vi "QMH_Tester_rev2.vi"() -> ()   [LabVIEW 2024]
doc: "Demonstrates the fundamentals of the Queued Message Handler design pattern in LabVIEW. A queued message handler, in its simplest form, is composed of two loops. The Event Handling Loop responds to user interface events by enqueuing \"messages\" on a message queue. These messages are dequeued in the Message Handling Loop. Note that the Message Handling Loop is also capable of sending messages to itself."
uses:
  Controls/Control_Stop.ctl
  Controls/Control_Unitherm Connect Disconnect Bool.ctl
  Controls/Control_M4X Connect Disconnect Bool.ctl
  Controls/Control_Fornax Connect Disconnect Bool.ctl
  Controls/Control_Unitherm Set Load Numeric.ctl
  Controls/Control_Unitherm Set Load Bool.ctl
  Controls/Control_Unitherm VISA Resource.ctl
  Controls/Control_Unitherm Clear Load Bool.ctl
  Controls/Control_PXI-7854R Connect Disconnect Bool.ctl
  Controls/Control_PXI-7854R 75kHz Bool.ctl
  Controls/Control_PXI-7854R uSec Off Numeric.ctl
  Controls/Control_PXI-7854R uSec On Numeric.ctl
  Controls/Control_PXI-7854R Resource.ctl
  Controls/Control_PXI-7854R Set Config Bool.ctl
  Controls/Control_PXI-7854R Set Config Enum.ctl
  Controls/Control_M4X Read Current Bool.ctl
  Controls/Control_Log Bool.ctl
  Controls/Control_Fornax Ligasure Activate Port Bool.ctl
  Controls/Control_Fornax Bipolar Activate Port Bool.ctl
  Controls/Control_Fornax Bipolar Decrease Power.ctl
  Controls/Control_Fornax Bipolar Increase Power.ctl
  Controls/Control_Fornax Bipolar Enum.ctl
  Controls/Control_Fornax Mono1 Cut Activate Port Bool.ctl
  Controls/Control_Fornax Mono1 Cut Enum.ctl
  Controls/Control_Fornax Mono1 Cut Increase Power.ctl
  Controls/Control_Fornax Mono1 Cut Decrease Power.ctl
  Controls/Control_Fornax Mono1 Coag Enum.ctl
  Controls/Control_Fornax Mono1 Coag Activate Port Bool.ctl
  Controls/Control_Fornax Mono1 Coag Increase Power.ctl
  Controls/Control_Fornax Mono1 Coag Decrease Power.ctl
  Controls/Control_Fornax Mono2 Cut Activate Port Bool.ctl
  Controls/Control_Fornax Mono2 Cut Increase Power.ctl
  Controls/Control_Fornax Mono2 Cut Decrease Power.ctl
  Controls/Control_Fornax Mono2 Cut Enum.ctl
  Controls/Control_Fornax Mono2 Coag Activate Port Bool.ctl
  Controls/Control_Fornax Mono2 Coag Enum.ctl
  Controls/Control_Fornax Mono2 Coag Increase Power.ctl
  Controls/Control_Fornax Mono2 Coag Decrease Power.ctl
  NI Online Practice/CLD Practice/cld_success_package/Preparation_Materials/CLD 6/CLD 6 CSV file enum.ctl
  Controls/Control_Semi-Auto 2-D Array.ctl
  Controls/Control_Fornax Mono1 Cut Power Indicator.ctl
  Controls/Control_Fornax Mono1 Coag Power Indicator.ctl
  Controls/Control_Fornax Mono2 Cut Power Indicator.ctl
  Controls/Control_Fornax Mono2 Coag Power Indicator.ctl
  Controls/Control_Fornax Bipolar Power Indicator.ctl
  Controls/Control_Semi-Auto Cluster Array.ctl
  Controls/Control_Semi-Auto Cluster.ctl
  Controls/Control_Semi-Auto Unitherm Load.ctl
  Controls/Control_Semi-Auto Port.ctl
  Controls/Control_Semi-Auto Mode.ctl
  Controls/Control_Semi-Auto Power Level.ctl
  Controls/Control_Semi-Auto Activation Duration.ctl
  Controls/Control_Footswitch Resource Name.ctl
  Controls/Control_Semi-Auto Cluster Array 2.ctl
  Controls/Control_Semi-Auto Cluster 2.ctl
  Controls/Control_Semi-Auto 2 Activation Method.ctl
  Controls/QMH Fundamentals - Message Cluster.ctl
  Controls/Config_Stop Notifier Enum.ctl
  Controls/Control_Log Cluster.ctl
  Controls/Control_Log Time.ctl
  Controls/Control_Log Waveform Cluster - Current.ctl
  Controls/Control_Log Analysis Cluster - Current.ctl
  Controls/Control_Log Activation Settings Cluster.ctl
  Controls/Control_Log Unitherm Load.ctl
  Controls/Control_Log Port.ctl
  Controls/Control_Log Mode.ctl
  Controls/Control_Log Power Level.ctl
  Controls/Control_Log Waveform Cluster - Diff Voltage.ctl
  Controls/Control_Log Analysis Cluster - Diff Voltage.ctl
  Controls/Control_Log Loop Cluster.ctl
  Controls/Control_Log TDMS Filename.ctl
  Controls/Control_Log t0.ctl
  Controls/Control_Serial Number.ctl
  Controls/Control_Message Handling Cluster.ctl
  Controls/Control_M4X Connection.ctl
  Controls/Control_PXI-7854R FPGA Reference.ctl
  Controls/Control_Config Cluster.ctl
  Controls/Control_Config Unitherm Port.ctl
  Controls/Control_Config Simulate Values.ctl
  Controls/Control_Config Fornax Connect Attempts.ctl
  Controls/Control_Log Queue.ctl
  Controls/Control_Log Flag.ctl
  Controls/Control_Log Port Mode Cluster.ctl
  Controls/Control_Indicator Cluster.ctl
  Controls/Control_Log Power Level Cluster.ctl
  Controls/Control_Log Mono1 Cut Power.ctl
  Controls/Control_Log Mono1 Coag Power.ctl
  Controls/Control_Log Mono2 Cut Power.ctl
  Controls/Control_Log Mono2 Coag Power.ctl
  Controls/Control_Log Bipolar Power.ctl
  Controls/Control_Footswitch Reset Device Bool.ctl
  <instrlib>/niSwitch/niSwitch.llb/niSwitch Topologies.ctl
  Controls/Control_Footswitch Simulate Bool.ctl
  Controls/Control_Unitherm Connect Disconnect Cluster.ctl
  Controls/Control_PXI-7854R Connect Disconnect Cluster.ctl
  Controls/Control_PXI-7854R Set Config Cluster.ctl
  Controls/Control_Auto Set Power Cluster.ctl
  VIs/Abort Auto Test Global.vi
  <vilib>/Utility/error.llb/Error Cluster From Error Code.vi
  <vilib>/ErrorRing/Error Ring.xnode
panel:
  in  "Stop Button":bool
  out "Display Message":string="\"Stop\" button pressed"
  out "Array":T1(array[cluster])
  out "Logging?":bool
  in  "Log?":T2
  out "Fornax Connected?":bool
  out "Unitherm Connected?":bool
  out "M4X Connected?":bool
  out "PXI-7854R Connected?":bool
  in  "Stop":T3
  out "Data":waveform(dbl)[](graph)
  in  "Tab Control":T4(tab)=enum."Semi-Auto"
  out "Mono2 - Coag Power":T5
  out "Mono2 - Cut Power":T6
  out "Mono1 - Coag Power":T7
  out "Mono1 - Cut Power":T8
  in  "Ligasure Activate":T9
  in  "Bipolar Activate":T10
  in  "Bipolar minus":T11
  in  "Bipolar plus":T12
  in  "Bipolar Enum":T13
  in  "Mono1 Cut Activate":T14
  in  "Mono1 Cut Enum":T15
  in  "Mono1 Cut plus":T16
  in  "Mono1 Cut minus":T17
  in  "Mono1 Coag Enum":T18=enum."Spray"
  in  "Mono1 Coag Activate":T19
  in  "Mono1 Coag plus":T20
  in  "Mono1 Coag minus":T21
  in  "Mono2 Cut Activate":T22
  in  "Mono2 Cut plus":T23
  in  "Mono2 Cut minus":T24
  in  "Mono2 Cut Enum":T25
  in  "Mono2 Coag Activate":T26
  in  "Mono2 Coag Enum":T27=enum."Spray"
  in  "Mono2 Coag plus":T28
  in  "Mono2 Coag minus":T29
  out "Bipolar Power":T30
  in  "Unitherm Connect/Disconnect":T31=TRUE
  in  "Load (Ohms)":T32
  in  "Set Load":T33
  in  "Unitherm Refnum in":T34="COM4"
  in  "Clear Load":T35
  in  "7854 Connect/Disconnect":T36=TRUE
  in  "75kHz":T37=TRUE
  in  "uSec Off":T38=6
  in  "uSec On":T39=7
  in  "resource name":T40="PXI1Slot6" caption="RIO Device"
  in  "7854 Set Config":T41
  in  "7854 Config Enum":T42=enum."Off"
  in  "M4X Connect/Disconnect":T43=TRUE
  in  "Fornax Connect/Disconnect":T44=TRUE
  in  "Read Current":T45
  in  "Abort Auto Test":bool
  in  "Update Semi-Auto":bool
  in  "Read/ Write":T46
  in  "Path":path=path "C:/Users/yearon2/OneDrive - Medtronic PLC/LV2015/LT10 Generator Sandbox/FT10_rev2/Semi-Auto Commands.csv"
  out "Semi-Auto 2-D Array out":T47
  in  "Run Semi-Auto Commands":bool
  in  "Semi-Auto Cluster in":T48 {"Power Level" format="%.1f"}
  out "Set Load Case":string="False Case"
  in  "Mono1 Cut - Handswitch":bool
  in  "Mono1 Coag - Handswitch":bool
  in  "Mono2 Triverse Tab":enum32{"Mono 2 - 2 Button", "Mono 2 - Triverse"}(tab)
  in  "Mono2 Cut - Handswitch":bool
  in  "Mono2 Coag - Handswitch":bool
  in  "Triverse Slide":i8(slide) scale=1.0..5.0
  in  "Mono2 Triverse - Handswitch Seal":bool
  in  "Mono2 Triverse - Handswitch Cut":bool
  in  "Mono2 Triverse - Handswitch Coag":bool
  in  "Ligasure - Coag Footswitch":bool
  in  "Ligasure - Cut Footswitch":bool
  in  "Ligasure - Seal Footswitch":bool
  in  "Ligasure - Bipolar Footswitch":bool
  in  "Mono1 Cut - Footswitch":bool
  in  "Mono1 Coag - Footswitch":bool
  in  "Mono2 Cut - Footswitch":bool
  in  "Mono2 Coag - Footswitch":bool
  in  "Bipolar - Footswitch":bool
  in  "Mono2 Triverse - Footswitch":bool
  in  "PXI-2565 resource name":T55="PXI1Slot7" caption="resource name"
  out "Connected?":bool
  in  "Path 2":path=path "C:/Users/yearon2/OneDrive - Medtronic PLC/LV2024/LT10 Generator Sandbox/FT10_rev2/Semi-Auto 2 Commands.csv"
  in  "Run Semi-Auto 2 Commands":bool
  in  "Update Semi-Auto 2":bool
  in  "Read/ Write 2":T46
  out "Semi-Auto 2-D Array out 2":T47
  in  "Semi-Auto 2 Cluster in":T56
  # "Note: If you are creating a LabVIEW application based on the Queued Message Handler design pattern, create a Queued Message Handler project from the File > Create Project dialog."
  # "Bipolar"
  # "Mono2"
  # "Mono1"
  # "Ligasure"
  # "Unitherm"
  # "PXI-7854R"
  # "Fornax"
  # "M4X"
  # "Mono1"
  # "Mono2"
  # "Bipolar"
  # "Ligasure"
  # "Mono1"
  # "Mono2"
  # "Bipolar"
  # "Ligasure"
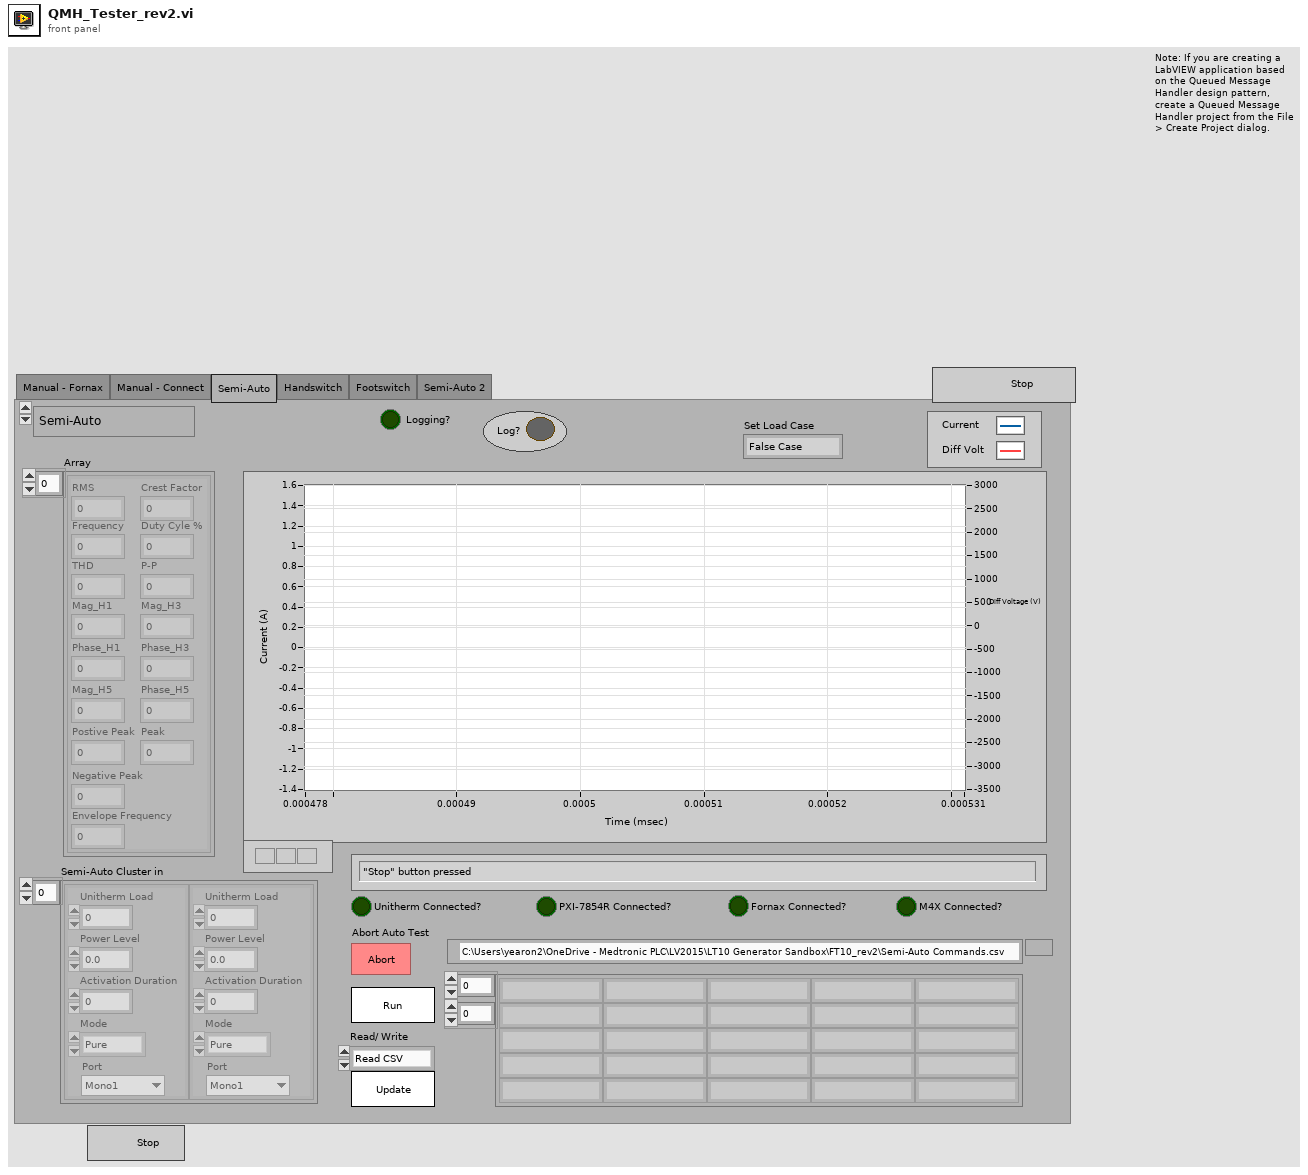
[diagram p1: front panel]
types:
  T1 = cluster{"RMS":dbl, "Envelope Frequency":dbl, "Peak":dbl, "Crest Factor":dbl, "Duty Cyle %":dbl, "P-P":dbl, "Frequency":dbl, "THD":dbl, "Postive Peak":dbl, "Negative Peak":dbl, "Mag_H1":dbl, "Phase_H1":dbl, "Mag_H3":dbl, "Phase_H3":dbl, "Mag_H5":dbl, "Phase_H5":dbl}[]
  T2 = typedef "Control_Log Bool.ctl" = bool
  T3 = typedef "Control_Stop.ctl" = bool
  T4 = enum32{"Manual - Fornax", "Manual - Connect", "Semi-Auto", "Handswitch", "Footswitch", "Semi-Auto 2"}
  T5 = typedef "Control_Fornax Mono2 Coag Power Indicator.ctl" = string
  T6 = typedef "Control_Fornax Mono2 Cut Power Indicator.ctl" = string
  T7 = typedef "Control_Fornax Mono1 Coag Power Indicator.ctl" = string
  T8 = typedef "Control_Fornax Mono1 Cut Power Indicator.ctl" = string
  T9 = typedef "Control_Fornax Ligasure Activate Port Bool.ctl" = bool
  T10 = typedef "Control_Fornax Bipolar Activate Port Bool.ctl" = bool
  T11 = typedef "Control_Fornax Bipolar Decrease Power.ctl" = bool
  T12 = typedef "Control_Fornax Bipolar Increase Power.ctl" = bool
  T13 = typedef "Control_Fornax Bipolar Enum.ctl" = enum16{"Standard", "Macro", "Precision"}
  T14 = typedef "Control_Fornax Mono1 Cut Activate Port Bool.ctl" = bool
  T15 = typedef "Control_Fornax Mono1 Cut Enum.ctl" = enum16{"Pure", "Blend"}
  T16 = typedef "Control_Fornax Mono1 Cut Increase Power.ctl" = bool
  T17 = typedef "Control_Fornax Mono1 Cut Decrease Power.ctl" = bool
  T18 = typedef "Control_Fornax Mono1 Coag Enum.ctl" = enum16{"Fulgerate", "Spray"}
  T19 = typedef "Control_Fornax Mono1 Coag Activate Port Bool.ctl" = bool
  T20 = typedef "Control_Fornax Mono1 Coag Increase Power.ctl" = bool
  T21 = typedef "Control_Fornax Mono1 Coag Decrease Power.ctl" = bool
  T22 = typedef "Control_Fornax Mono2 Cut Activate Port Bool.ctl" = bool
  T23 = typedef "Control_Fornax Mono2 Cut Increase Power.ctl" = bool
  T24 = typedef "Control_Fornax Mono2 Cut Decrease Power.ctl" = bool
  T25 = typedef "Control_Fornax Mono2 Cut Enum.ctl" = enum16{"Pure", "Blend"}
  T26 = typedef "Control_Fornax Mono2 Coag Activate Port Bool.ctl" = bool
  T27 = typedef "Control_Fornax Mono2 Coag Enum.ctl" = enum16{"Fulgerate", "Spray"}
  T28 = typedef "Control_Fornax Mono2 Coag Increase Power.ctl" = bool
  T29 = typedef "Control_Fornax Mono2 Coag Decrease Power.ctl" = bool
  T30 = typedef "Control_Fornax Bipolar Power Indicator.ctl" = string
  T31 = typedef "Control_Unitherm Connect Disconnect Bool.ctl" = bool
  T32 = typedef "Control_Unitherm Set Load Numeric.ctl" = i32
  T33 = typedef "Control_Unitherm Set Load Bool.ctl" = bool
  T34 = typedef "Control_Unitherm VISA Resource.ctl" = refnum<visa-resource-name>
  T35 = typedef "Control_Unitherm Clear Load Bool.ctl" = bool
  T36 = typedef "Control_PXI-7854R Connect Disconnect Bool.ctl" = bool
  T37 = typedef "Control_PXI-7854R 75kHz Bool.ctl" = bool
  T38 = typedef "Control_PXI-7854R uSec Off Numeric.ctl" = u16
  T39 = typedef "Control_PXI-7854R uSec On Numeric.ctl" = u16
  T40 = typedef "Control_PXI-7854R Resource.ctl" = tag
  T41 = typedef "Control_PXI-7854R Set Config Bool.ctl" = bool
  T42 = typedef "Control_PXI-7854R Set Config Enum.ctl" = enum16{"Mono 1", "Mono 2", "BiPolar", "LigaSure", "Off"}
  T43 = typedef "Control_M4X Connect Disconnect Bool.ctl" = bool
  T44 = typedef "Control_Fornax Connect Disconnect Bool.ctl" = bool
  T45 = typedef "Control_M4X Read Current Bool.ctl" = bool
  T46 = typedef "CLD 6 CSV file enum.ctl" = enum16{"Read CSV", "Write CSV"}
  T47 = typedef "Control_Semi-Auto 2-D Array.ctl" = string[][]
  T48 = typedef "Control_Semi-Auto Cluster Array.ctl" = T49[]
  T49 = typedef "Control_Semi-Auto Cluster.ctl" = cluster{"Unitherm Load":T50, "Port":T51, "Mode":T52, "Power Level":T53, "Activation Duration":T54}
  T50 = typedef "Control_Semi-Auto Unitherm Load.ctl" = i32
  T51 = typedef "Control_Semi-Auto Port.ctl" = enum16{"Mono1", "Mono2", "Bipolar", "Ligasure", "Error"}
  T52 = typedef "Control_Semi-Auto Mode.ctl" = enum16{"Pure", "Blend", "Spray", "Fulgerate", "Standard", "Macro", "Precision", "Ligasure", "Error"}
  T53 = typedef "Control_Semi-Auto Power Level.ctl" = dbl
  T54 = typedef "Control_Semi-Auto Activation Duration.ctl" = i32
  T55 = typedef "Control_Footswitch Resource Name.ctl" = refnum<k15>
  T56 = typedef "Control_Semi-Auto Cluster Array 2.ctl" = T57[]
  T57 = typedef "Control_Semi-Auto Cluster 2.ctl" = cluster{"Mode":T52, "Unitherm Load":T50, "Power Level":T53, "Activation Duration":T54, "Port":T51, "Activation Method":T58}
  T58 = typedef "Control_Semi-Auto 2 Activation Method.ctl" = enum16{"Fornax", "Handswitch", "Footswitch"}
  T59 = typedef "Control_Log Loop Cluster.ctl" = cluster{"tdms file out":T60, "t0":T61, "Generator Serial Number in":T62}
  T60 = typedef "Control_Log TDMS Filename.ctl" = refnum<k34>
  T61 = typedef "Control_Log t0.ctl" = string
  T62 = typedef "Control_Serial Number.ctl" = string
  T63 = typedef "Config_Stop Notifier Enum.ctl" = enum16{"Initialize", "Read Notifier", "Notify", "Close"}
  T64 = typedef "Control_Log Cluster.ctl" = cluster{"Log Time":T65, "Log Waveform Cluster - Current":T66, "Log Analysis Cluster - Current":T67, "Log - Activation Settings Cluster":T68, "Log Waveform Cluster - Diff Voltage":T73, "Log Analysis Cluster - Diff Voltage":T74}
  T65 = typedef "Control_Log Time.ctl" = timestamp
  T66 = typedef "Control_Log Waveform Cluster - Current.ctl" = waveform(dbl)
  T67 = typedef "Control_Log Analysis Cluster - Current.ctl" = cluster{"RMS":dbl, "Envelope Frequency":dbl, "Peak":dbl, "Crest Factor":dbl, "Duty Cyle %":dbl, "P-P":dbl, "Frequency":dbl, "THD":dbl, "Postive Peak":dbl, "Negative Peak":dbl, "Mag_H1":dbl, "Phase_H1":dbl, "Mag_H3":dbl, "Phase_H3":dbl, "Mag_H5":dbl, "Phase_H5":dbl}
  T68 = typedef "Control_Log Activation Settings Cluster.ctl" = cluster{"Log - Unitherm Load":T69, "Log - Port":T70, "Log - Mode":T71, "Log - Power Level":T72}
  T69 = typedef "Control_Log Unitherm Load.ctl" = string
  T70 = typedef "Control_Log Port.ctl" = string
  T71 = typedef "Control_Log Mode.ctl" = string
  T72 = typedef "Control_Log Power Level.ctl" = string
  T73 = typedef "Control_Log Waveform Cluster - Diff Voltage.ctl" = waveform(dbl)
  T74 = typedef "Control_Log Analysis Cluster - Diff Voltage.ctl" = cluster{"RMS":dbl, "Envelope Frequency":dbl, "Peak":dbl, "Crest Factor":dbl, "Duty Cyle %":dbl, "P-P":dbl, "Frequency":dbl, "THD":dbl, "Postive Peak":dbl, "Negative Peak":dbl, "Mag_H1":dbl, "Phase_H1":dbl, "Mag_H3":dbl, "Phase_H3":dbl, "Mag_H5":dbl, "Phase_H5":dbl}
  T75 = typedef "QMH Fundamentals - Message Cluster.ctl" = cluster{"Message":string, "Message Data":variant}
  T76 = typedef "Control_Footswitch Simulate Bool.ctl" = bool
  T77 = typedef "niSwitch Topologies.ctl" = string
  T78 = typedef "Control_Footswitch Reset Device Bool.ctl" = bool
  T79 = typedef "Control_Message Handling Cluster.ctl" = cluster{"Fornax Connected?":refnum<vi>, "Unitherm Connected?":refnum<vi>, "M4X Connected?":refnum<vi>, "Unitherm Connect/Disconnect":refnum<vi>, "Fornax Connection":refnum<k5>, "UNITHERM Connection":refnum<visa-resource-name>, "M4X Connection":T80, "FPGA VI Reference Out":T81, "PXI-7854R Connected?":refnum<vi>, "Fornax Connect/Disconnect":refnum<vi>, "7854 Connect/Disconnect":refnum<vi>, "M4X Connect/Disconnect":refnum<vi>, "Config cluster":T82, "Log Queue":T86, "Log Analysis Cluster - Current":T67, "Log Waveform Cluster - Current":T66, "Log Time":T65, "Log Flag":T87, "Log - Activation Settings Cluster":T68, "Log - Port Mode Cluster":T88, "Log Analysis Cluster - Diff Voltage":T74, "Log Waveform Cluster - Diff Voltage":T73, "Indicator Cluster":T89, "Log Power Level Cluster":T90, "Footswitch Cluster":cluster{"PXI-2565 reset device (boolean value)":T78, "topology name":T77, "PXI-2565 simulate (boolean value)":T76, "PXI-2565 resource name":T55}}
  T80 = typedef "Control_M4X Connection.ctl" = u32
  T81 = typedef "Control_PXI-7854R FPGA Reference.ctl" = refnum<k20>
  T82 = typedef "Control_Config Cluster.ctl" = cluster{"Unitherm Port":T83, "Simulate Values":T84, "Fornax Connect Attempts":T85}
  T83 = typedef "Control_Config Unitherm Port.ctl" = string
  T84 = typedef "Control_Config Simulate Values.ctl" = bool
  T85 = typedef "Control_Config Fornax Connect Attempts.ctl" = i32
  T86 = typedef "Control_Log Queue.ctl" = refnum<queue>
  T87 = typedef "Control_Log Flag.ctl" = bool
  T88 = typedef "Control_Log Port Mode Cluster.ctl" = cluster{"Mono1 Cut Enum":T15, "Mono2 Cut Enum":T25, "Mono1 Coag Enum":T18, "Mono2 Coag Enum":T27, "Bipolar Enum":T13}
  T89 = typedef "Control_Indicator Cluster.ctl" = cluster{"Mono1 - Cut Power":refnum<vi>, "Mono1 - Coag Power":refnum<vi>, "Mono2 - Cut Power":refnum<vi>, "Mono2 - Coag Power":refnum<vi>, "Bipolar Power":refnum<vi>, "Mono1 Cut Enum":refnum<vi>, "Mono1 Coag Enum":refnum<vi>, "Mono2 Cut Enum":refnum<vi>, "Mono2 Coag Enum":refnum<vi>, "Bipolar Enum":refnum<vi>}
  T90 = typedef "Control_Log Power Level Cluster.ctl" = cluster{"Log Mono1 Cut Power":T91, "Log Mono1 Coag Power":T92, "Log Mono2 Cut Power":T93, "Log Mono2 Coag Power":T94, "Log Bipolar Power":T95}
  T91 = typedef "Control_Log Mono1 Cut Power.ctl" = string
  T92 = typedef "Control_Log Mono1 Coag Power.ctl" = string
  T93 = typedef "Control_Log Mono2 Cut Power.ctl" = string
  T94 = typedef "Control_Log Mono2 Coag Power.ctl" = string
  T95 = typedef "Control_Log Bipolar Power.ctl" = string
  T96 = typedef "Control_Unitherm Connect Disconnect Cluster.ctl" = cluster{"Unitherm Connect/Disconnect":T31, "Unitherm Refnum in":T34}
  T97 = typedef "Control_PXI-7854R Connect Disconnect Cluster.ctl" = cluster{"PXI-7854R Resource":T40, "75kHz":T37, "uSec Off":T38, "uSec On":T39, "7854 Connect/Disconnect":T36}
  T98 = typedef "Control_PXI-7854R Set Config Cluster.ctl" = cluster{"7854 Config Enum":T42, "7854 Set Config":T41}
  T99 = enum16{"Off", "Mono1 Relay Config", "Mono2 Relay Config", "Bipolar Relay Config", "Ligasure Relay Config", "Handswitch - Mono1 Cut", "Handswitch - Mono1 Coag", "Handswitch - Mono2 Cut", "Handswitch - Mono2 Coag", "Switch to Triverse Mode", "Switch to Mono2 - 2 button Mode", "Triverse Power 1", "Triverse Power 2", "Triverse Power 3", "Triverse Power 4", "Triverse Power 5", "Handswitch - Triverse Seal", "Handswitch - Triverse Cut", "Handswitch - Triverse Coag"}
  T100 = typedef "Control_Auto Set Power Cluster.ctl" = cluster{"Port":T51, "Mode":T52, "Power Level":T53}
  T101 = typedef "Control_Log Filename Cluster.ctl" = cluster{"Current Wvfrm filename":string, "Diff Volt Wvfrm filename":string}
  T102 = typedef "Control_Command Cluster.ctl" = cluster{"Message":string, "Message Data":variant, "Wait Time (ms)":i32}
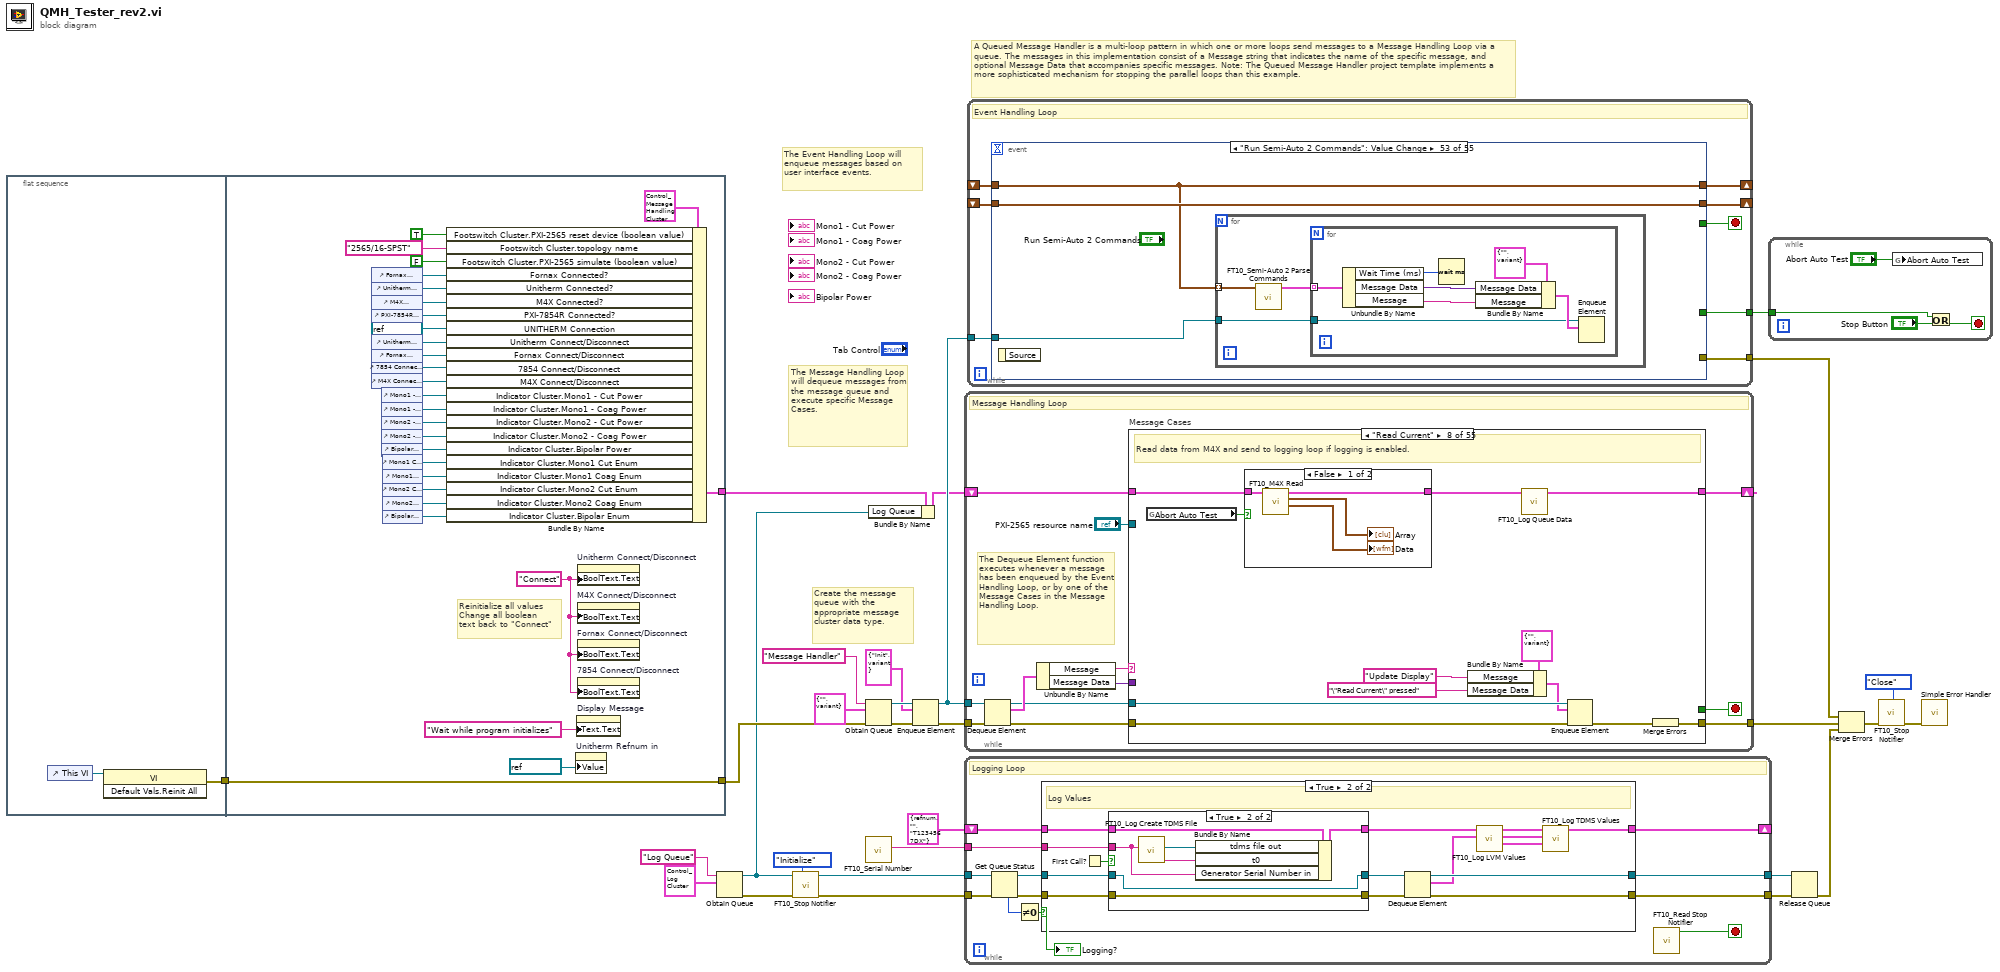
[diagram p0: block diagram]
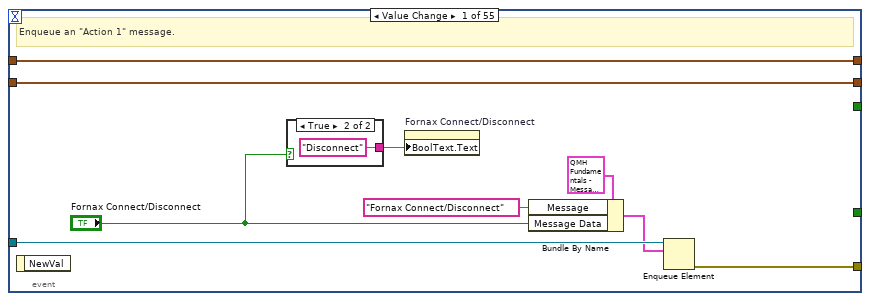
[diagram p4: hidden frame]
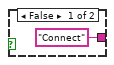
[diagram p5: hidden frame]
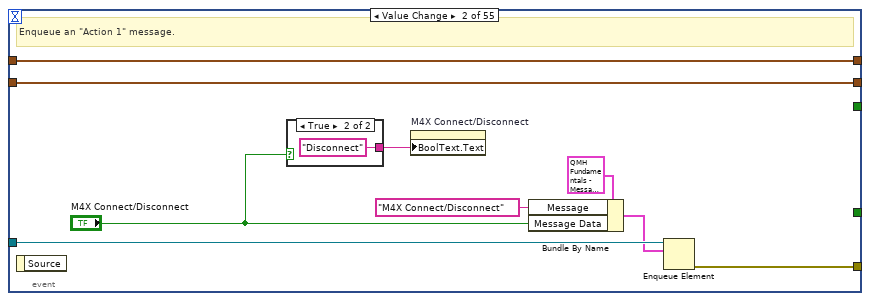
[diagram p6: hidden frame]
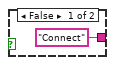
[diagram p7: hidden frame]
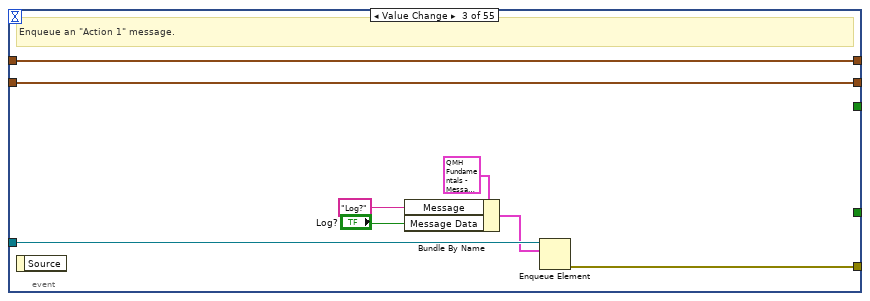
[diagram p8: hidden frame]
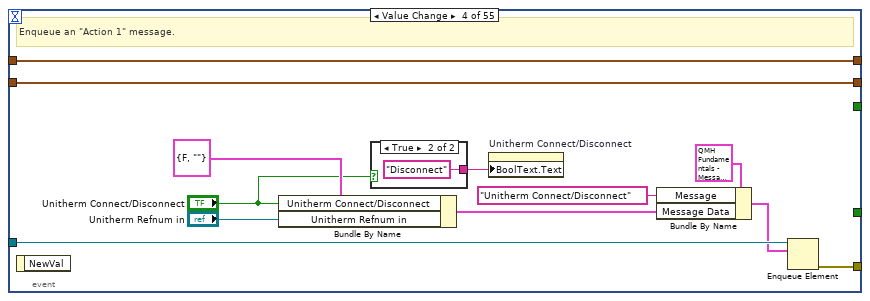
[diagram p9: hidden frame]
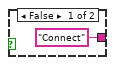
[diagram p10: hidden frame]
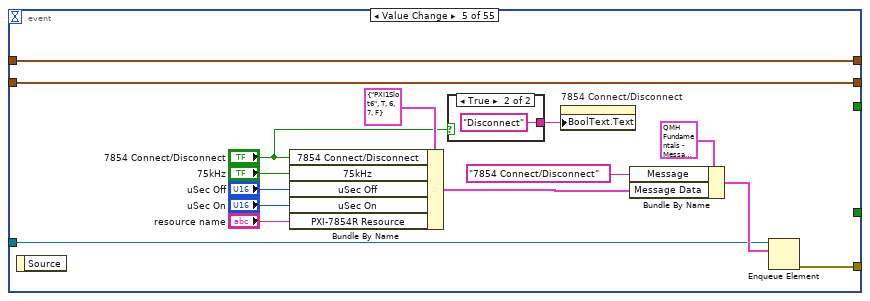
[diagram p11: hidden frame]
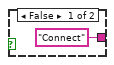
[diagram p12: hidden frame]
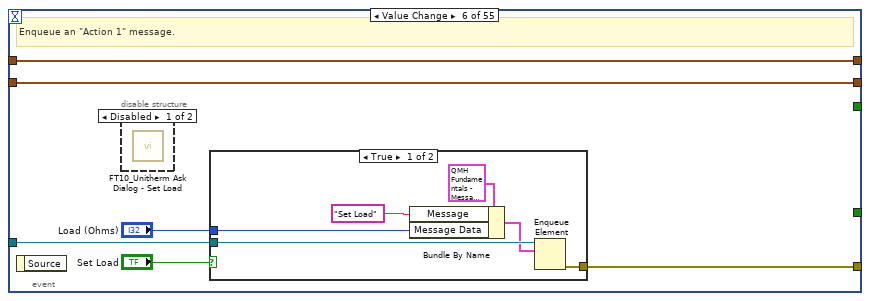
[diagram p13: hidden frame]
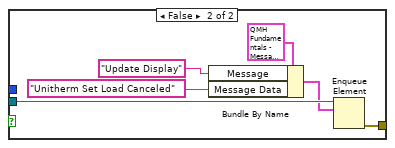
[diagram p15: hidden frame]
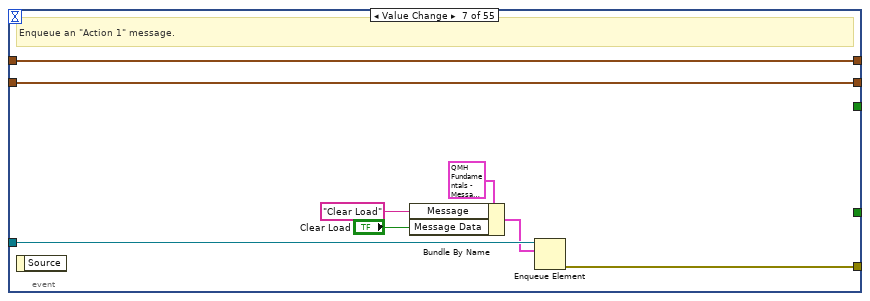
[diagram p16: hidden frame]
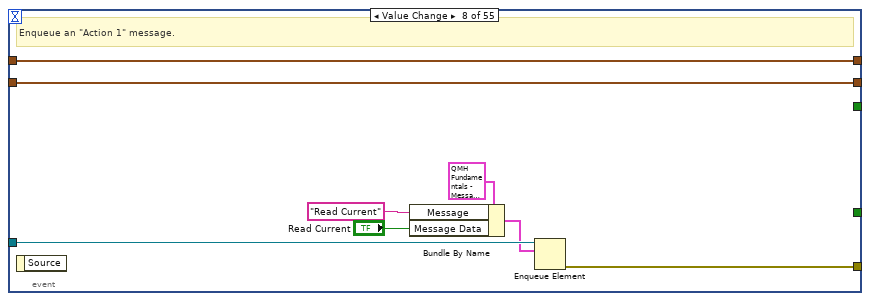
[diagram p17: hidden frame]
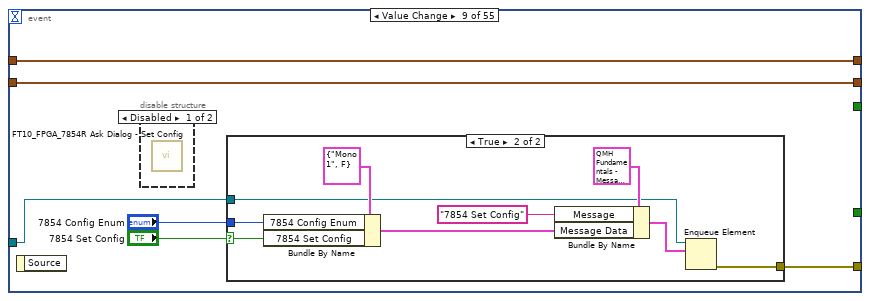
[diagram p18: hidden frame]
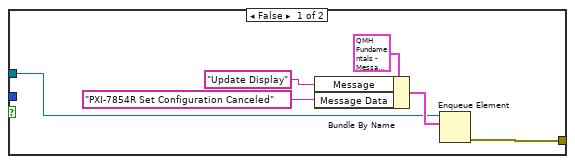
[diagram p20: hidden frame]
diagram:
  # "Create the message queue with the appropriate message cluster data type."
  # "A Queued Message Handler is a multi-loop pattern in which one or more loops send messages to a Message Handling Loop via a queue. The messages in this implementation consist of a Message string that indicates the name of the specific message, and optional Message Data that accompanies specific messages. Note: The Queued Message Handler project template implements a more sophisticated mechanism for stopping the parallel loops than this example."
  # "The Message Handling Loop will dequeue messages from the message queue and execute specific Message Cases."
  # "The Event Handling Loop will enqueue messages based on user interface events."
  n1 = flat-sequence {
    tunnel: [w29] -> w18
    tunnel: [w58] -> w21
    tunnel: w18 -> [w58]
    tunnel: [w48] -> w4
    frame #0 {
      n2 = control-ref of="This VI"() -> (w30:refnum<vi>)
      n3 = invoke class="VI" method="Default Vals.Reinit All"(reference=w30) -> (error out=w29:errorcluster)  [unwired: 2 in, 2 out]
    }
    frame #1 {
      w56 = "Connect" ("Boolean Text.Text")
      # "Reinitialize all values\nChange all boolean\ntext back to \"Connect\""
      n4 = control-ref of="Fornax Connected?"() -> (w34:refnum<vi>)
      n5 = control-ref of="Unitherm Connected?"() -> (w35:refnum<vi>)
      n6 = control-ref of="M4X Connected?"() -> (w36:refnum<vi>)
      n7 = control-ref of="PXI-7854R Connected?"() -> (w37:refnum<vi>)
      n8 = control-ref of="Unitherm Connect/Disconnect"() -> (w39:refnum<vi>)
      n9 = control-ref of="Fornax Connect/Disconnect"() -> (w40:refnum<vi>)
      n10 = control-ref of="7854 Connect/Disconnect"() -> (w41:refnum<vi>)
      n11 = control-ref of="M4X Connect/Disconnect"() -> (w42:refnum<vi>)
      n12 = control-ref of="Mono1 - Cut Power"() -> (w53:refnum<vi>)
      n13 = control-ref of="Mono1 - Coag Power"() -> (w52:refnum<vi>)
      n14 = control-ref of="Mono2 - Cut Power"() -> (w51:refnum<vi>)
      n15 = control-ref of="Mono2 - Coag Power"() -> (w50:refnum<vi>)
      n16 = control-ref of="Bipolar Power"() -> (w49:refnum<vi>)
      n17 = control-ref of="Mono1 Cut Enum"() -> (w47:refnum<vi>)
      n18 = control-ref of="Mono1 Coag Enum"() -> (w46:refnum<vi>)
      n19 = control-ref of="Mono2 Cut Enum"() -> (w45:refnum<vi>)
      n20 = control-ref of="Mono2 Coag Enum"() -> (w44:refnum<vi>)
      n21 = control-ref of="Bipolar Enum"() -> (w43:refnum<vi>)
      n22 = Bundle By Name(cluster=T79 {"Fornax Connected?"=refnum, "Unitherm Connected?"=refnum, "M4X Connected?"=refnum, "Unitherm Connect/Disconnect"=refnum, "Fornax Connection"=refnum, "UNITHERM Connection"="", "M4X Connection"=0, "FPGA VI Reference Out"=refnum, "PXI-7854R Connected?"=refnum, "Fornax Connect/Disconnect"=refnum, "7854 Connect/Disconnect"=refnum, "M4X Connect/Disconnect"=refnum, "Config cluster"={"Unitherm Port"="COM4", "Simulate Values"=TRUE, "Fornax Connect Attempts"=0}, "Log Queue"=refnum, "Log Analysis Cluster - Current"={"RMS"=0.0, "Envelope Frequency"=0.0, "Peak"=0.0, "Crest Factor"=0.0, "Duty Cyle %"=0.0, "P-P"=0.0, "Frequency"=0.0, "THD"=0.0, "Postive Peak"=0.0, "Negative Peak"=0.0, "Mag_H1"=0.0, "Phase_H1"=0.0, "Mag_H3"=0.0, "Phase_H3"=0.0, "Mag_H5"=0.0, "Phase_H5"=0.0}, "Log Waveform Cluster - Current"={"t0"=timestamp(0 s since 1904-01-01), "dt"=1.0, "Y"=[]}, "Log Time"=timestamp(0 s since 1904-01-01), "Log Flag"=FALSE, "Log - Activation Settings Cluster"={"Log - Unitherm Load"="", "Log - Port"="", "Log - Mode"="", "Log - Power Level"=""}, "Log - Port Mode Cluster"={"Mono1 Cut Enum"=enum."Pure", "Mono2 Cut Enum"=enum."Pure", "Mono1 Coag Enum"=enum."Spray", "Mono2 Coag Enum"=enum."Spray", "Bipolar Enum"=enum."Standard"}, "Log Analysis Cluster - Diff Voltage"={"RMS"=0.0, "Envelope Frequency"=0.0, "Peak"=0.0, "Crest Factor"=0.0, "Duty Cyle %"=0.0, "P-P"=0.0, "Frequency"=0.0, "THD"=0.0, "Postive Peak"=0.0, "Negative Peak"=0.0, "Mag_H1"=0.0, "Phase_H1"=0.0, "Mag_H3"=0.0, "Phase_H3"=0.0, "Mag_H5"=0.0, "Phase_H5"=0.0}, "Log Waveform Cluster - Diff Voltage"={"t0"=timestamp(0 s since 1904-01-01), "dt"=1.0, "Y"=[]}, "Indicator Cluster"={"Mono1 - Cut Power"=refnum, "Mono1 - Coag Power"=refnum, "Mono2 - Cut Power"=refnum, "Mono2 - Coag Power"=refnum, "Bipolar Power"=refnum, "Mono1 Cut Enum"=refnum, "Mono1 Coag Enum"=refnum, "Mono2 Cut Enum"=refnum, "Mono2 Coag Enum"=refnum, "Bipolar Enum"=refnum}, "Log Power Level Cluster"={"Log Mono1 Cut Power"="", "Log Mono1 Coag Power"="", "Log Mono2 Cut Power"="", "Log Mono2 Coag Power"="", "Log Bipolar Power"=""}, "Footswitch Cluster"={"PXI-2565 reset device (boolean value)"=TRUE, "topology name"="2565/16-SPST", "PXI-2565 simulate (boolean value)"=FALSE, "PXI-2565 resource name"=""}}, "Footswitch Cluster.PXI-2565 reset device (boolean value)"=T78 TRUE, "Footswitch Cluster.topology name"=T77 "2565/16-SPST", "Footswitch Cluster.PXI-2565 simulate (boolean value)"=T76 FALSE, "Fornax Connected?"=w34, "Unitherm Connected?"=w35, "M4X Connected?"=w36, "PXI-7854R Connected?"=w37, "UNITHERM Connection"=refnum<visa-resource-name> "COM4", "Unitherm Connect/Disconnect"=w39, "Fornax Connect/Disconnect"=w40, "7854 Connect/Disconnect"=w41, "M4X Connect/Disconnect"=w42, "Indicator Cluster.Mono1 - Cut Power"=w53, "Indicator Cluster.Mono1 - Coag Power"=w52, "Indicator Cluster.Mono2 - Cut Power"=w51, "Indicator Cluster.Mono2 - Coag Power"=w50, "Indicator Cluster.Bipolar Power"=w49, "Indicator Cluster.Mono1 Cut Enum"=w47, "Indicator Cluster.Mono1 Coag Enum"=w46, "Indicator Cluster.Mono2 Cut Enum"=w45, "Indicator Cluster.Mono2 Coag Enum"=w44, "Indicator Cluster.Bipolar Enum"=w43) -> (w48:T79)
      n23 = property on="Unitherm Refnum in" class="VISAName (strict)"("Value"=refnum<visa-resource-name> "COM4" ("Unitherm Refnum in")) -> ()  [unwired: 2 in, 2 out]
      n24 = property on="Display Message" class="Str"("Text.Text"="Wait while program initializes" ("Display Message")) -> ()  [unwired: 2 in, 2 out]
      n25 = property on="Unitherm Connect/Disconnect" class="Bool (strict)"("BoolText.Text"=w56) -> ()  [unwired: 2 in, 2 out]
      n26 = property on="M4X Connect/Disconnect" class="Bool (strict)"("BoolText.Text"=w56) -> ()  [unwired: 2 in, 2 out]
      n27 = property on="Fornax Connect/Disconnect" class="Bool (strict)"("BoolText.Text"=w56) -> ()  [unwired: 2 in, 2 out]
      n28 = property on="7854 Connect/Disconnect" class="Bool (strict)"("BoolText.Text"=w56) -> ()  [unwired: 2 in, 2 out]
    }
  }
  n29 = Obtain Queue(name (unnamed)="Log Queue", element data type=T64 {"Log Time"=timestamp(0 s since 1904-01-01), "Log Waveform Cluster - Current"={"t0"=timestamp(0 s since 1904-01-01), "dt"=1.0, "Y"=[]}, "Log Analysis Cluster - Current"={"RMS"=0.0, "Envelope Frequency"=0.0, "Peak"=0.0, "Crest Factor"=0.0, "Duty Cyle %"=0.0, "P-P"=0.0, "Frequency"=0.0, "THD"=0.0, "Postive Peak"=0.0, "Negative Peak"=0.0, "Mag_H1"=0.0, "Phase_H1"=0.0, "Mag_H3"=0.0, "Phase_H3"=0.0, "Mag_H5"=0.0, "Phase_H5"=0.0}, "Log - Activation Settings Cluster"={"Log - Unitherm Load"="", "Log - Port"="", "Log - Mode"="", "Log - Power Level"=""}, "Log Waveform Cluster - Diff Voltage"={"t0"=timestamp(0 s since 1904-01-01), "dt"=1.0, "Y"=[]}, "Log Analysis Cluster - Diff Voltage"={"RMS"=0.0, "Envelope Frequency"=0.0, "Peak"=0.0, "Crest Factor"=0.0, "Duty Cyle %"=0.0, "P-P"=0.0, "Frequency"=0.0, "THD"=0.0, "Postive Peak"=0.0, "Negative Peak"=0.0, "Mag_H1"=0.0, "Phase_H1"=0.0, "Mag_H3"=0.0, "Phase_H3"=0.0, "Mag_H5"=0.0, "Phase_H5"=0.0}}) -> (queue out=w11:refnum<queue>, error out=w9:errorcluster)  [unwired: 3 in, 1 out]
  n30 = call "FT10_Stop Notifier.vi"("Selector"=Config_Stop_Notifier_Enum."Initialize", "error in (no error)"=w9) -> ("error out"=w8:errorcluster)  [unwired: 8 in, 1 out]
  n31 = call "FT10_Serial Number.vi"() -> ("Generator Serial Number out"=w2:T62)  [unwired: 11 in]
  n32 = Obtain Queue(name (unnamed)="Message Handler", element data type=T75 {"Message"="", "Message Data"=variant} ("Message Cluster"), error in (no error)=w21) -> (queue out=w24:refnum<queue>, error out=w25:errorcluster)  [unwired: 2 in, 1 out]
  n33 = Bundle By Name(cluster=w4, "Log Queue"=w11) -> (w12:T79)
  n34 = Enqueue Element(queue=w24, element=T75 {"Message"="Init", "Message Data"=variant}, error in (no error)=w25) -> (queue out=w19:refnum<queue>, error out=w23:errorcluster)  [unwired: 1 in, 1 out]
  n35 = while {
    tunnel: w19 -> [w69]
    tunnel: w23 -> [w70]
    tunnel: [w62] -> w28
    shift-right: [w63] -> _
    shift-left: w12 -> [w60]
    stop <- w61 stop-if-true
    # "The Dequeue Element function executes whenever a message has been enqueued by the Event Handling Loop, or by one of the Message Cases in the Message Handling Loop."
    # "Message Handling Loop"
    n36 = Dequeue Element(queue=w69, error in (no error)=w70) -> (queue out=w67:refnum<queue>, element=w68:T75, error out=w66:errorcluster)  [unwired: 1 in, 1 out]
    n37 = Unbundle By Name(w68) -> ("Message"=w65:string, "Message Data"=w64:variant)
    n38 = case "Message Cases" shown="\"Read Current\"" w65 {
      selector: w65 -> [_ _ _ _ _ _ _ _ _ _ _ _ _ _ _ _ _ _ _ _ _ _ _ _ _ _ _ _ _ _ _ _ _ _ _ _ _ _ _ _ _ _ _ _ _ _ _ _ _ _ _ _ _ _ w994]
      tunnel: w67 -> [w83 w100 w119 w148 w167 w195 w210 w222 w230 w267 w288 w303 w318 w333 w348 w363 w373 w390 w407 w424 w441 w458 w478 w495 w512 w538 w559 w580 w601 w622 w643 w664 w685 w706 w727 w739 w749 w759 w769 w779 w789 w799 w809 w819 w829 w845 w868 w891 w914 w937 w954 _ _ w988 _]
      tunnel: w66 -> [w71 w99 w110 w139 w158 w182 w200 w214 w233 w268 w287 w302 w317 w332 w347 w362 w375 w392 w409 w426 w443 w460 w480 w497 w514 w533 w554 w575 w596 w617 w638 w659 w680 w701 w722 w738 w748 w758 w768 w778 w788 w798 w808 w818 w828 w844 w867 w890 w913 w936 w953 w967 w973 w981 w993]
      tunnel: [w84 w101 w120 w149 w168 w188 w204 w216 w234 w269 w286 w301 w316 w331 w346 w361 w376 w393 w410 w427 w444 w461 w481 w498 w515 w540 w561 w582 w603 w624 w645 w666 w687 w708 w729 w737 w747 w757 w767 w777 w787 w797 w807 w817 w827 w843 w866 w889 w912 w935 w952 w967 w970 w978 w993] -> w62
      tunnel: w64 -> [_ w94 w117 w138 w159 w186 _ _ w239 w273 w283 w299 w314 w328 w343 w358 w380 w397 w414 w431 w448 w465 w485 w502 w519 w544 w565 w586 w607 w628 w649 w670 w691 w712 w733 _ _ _ _ _ _ _ _ _ _ w840 w862 w885 w908 w931 w951 w966 w972 _ _]
      tunnel: w60 -> [w82 w105 w112 w143 w161 w189 w205 w217 w241 w264 w285 w300 w315 w330 w345 w360 w382 w399 w416 w433 w450 w467 w487 w504 w521 w536 w557 w578 w599 w620 w641 w662 w683 w704 w725 w736 w746 w756 w766 w776 w786 w796 w806 w816 w826 w842 w865 w888 w911 w934 w950 w965 w968 w983 w991]
      tunnel: [w80 w98 w111 w142 w160 w176 w197 w212 w240 w262 w279 w294 w309 w324 w339 w354 w381 w398 w415 w432 w449 w466 w486 w503 w520 w530 w551 w572 w593 w614 w635 w656 w677 w698 w719 w735 w745 w754 w764 w774 w784 w794 w804 w814 w824 w836 w859 w882 w905 w928 w950 w964 w968 w982 w991] -> w63
      tunnel: [_ _ _ _ _ _ _ _ _ _ _ _ _ _ _ _ _ _ _ _ _ _ _ _ _ _ _ _ _ _ _ _ _ _ _ _ _ _ _ _ _ _ _ _ _ _ _ _ _ _ _ _ _ TRUE _] -> w61
      tunnel: "PXI-2565 resource name" -> [_ _ _ _ _ _ _ _ _ _ _ _ _ _ _ _ _ _ _ _ _ _ _ _ _ w535 w556 w577 w598 w619 w640 w661 w682 w703 w724 _ _ _ _ _ _ _ _ _ _ _ _ _ _ _ _ _ _ _ _]
      frame "Init" {
        # "Initialize - Create reference for connection indicators. Connect to Fornax, M4X, and Unitherm."
        n39 = call "FT10_Config Parse File.vi"("error in (no error)"=w71, "File Path Control"=path "Config.ini") -> ("error out"=w73:errorcluster, "Config cluster"=w72:T82)  [unwired: 8 in]
        n40 = Bundle By Name(cluster=w82, "Config cluster"=w72) -> (w81:T79)
        n41 = Bundle By Name(cluster=T75 {"Message"="", "Message Data"=variant} ("Message Cluster"), "Message"="Update Display", "Message Data"="Initialize Complete" ("L10n_Action 1 Pressed")) -> (w87:T75)
        n42 = call "FT10_Connect Hardware.vi"("Message Handling Cluster in"=w81, "error in (no error)"=w73) -> ("Message Handling Cluster out"=w80:T79, "Fornax Connected?"=→"Fornax Connected?":bool, "Unitherm Connected?"=→"Unitherm Connected?":bool, "M4X Connected?"=→"M4X Connected?":bool, "PXI-7854R Connected?"=→"PXI-7854R Connected?":bool, "error out"=w79:errorcluster)  [unwired: 8 in]
        n43 = Enqueue Element(queue=w83, element=w87, error in (no error)=w71) -> (error out=w85:errorcluster)  [unwired: 1 in, 2 out]
        n44 = Merge Errors(w79, w85) -> (w84:errorcluster)
      }
      frame "Fornax Connect/Disconnect" {
        # "Connect or disconnect from Fornax."
        n45 = Variant To Data(type=TRUE, Variant=w94) -> (data=w91:bool)  [unwired: 1 in, 1 out]
        n46 = case shown="True" w91 {
          tunnel: ["Fornax Disconnect" ("L10n_Action 1 Pressed") "Fornax Connect" ("L10n_Action 1 Pressed")] -> w90
          frame False {
          }
          frame True {
          }
        }
        n47 = call "FT10_Connect Fornax Handler.vi"("error in (no error)"=w99, "Message Data"=w94, "Message Handling Cluster in"=w105) -> ("error out"=w96:errorcluster, "Fornax Connected?"=w95:bool, "Message Handling Cluster out"=w98:T79)  [unwired: 6 in]
        n48 = Bundle By Name(cluster=T75 {"Message"="", "Message Data"=variant} ("Message Cluster"), "Message Data"=w90, "Message"="Update Display") -> (w103:T75)
        n49 = Enqueue Element(queue=w100, element=w103, error in (no error)=w99) -> (error out=w102:errorcluster)  [unwired: 1 in, 2 out]
        n50 = Unbundle By Name(w98) -> ("Fornax Connected?"=w97:refnum<vi>)
        n51 = property class="Bool (strict)"(reference=w97, "Value"=w95) -> ()  [unwired: 1 in, 2 out]
        n52 = Merge Errors(w96, w102) -> (w101:errorcluster)
      }
      frame "M4X Connect/Disconnect" {
        # "Connect or disconnect from M4X."
        n53 = Variant To Data(type=TRUE, Variant=w117) -> (data=w114:bool)  [unwired: 1 in, 1 out]
        n54 = case shown="True" w114 {
          tunnel: ["M4X Disconnect" ("L10n_Action 1 Pressed") "M4X Connect" ("L10n_Action 1 Pressed")] -> w113
          tunnel: w112 -> [w126 w132]
          tunnel: [w126 w131] -> w111
          tunnel: w110 -> [w125 w130]
          tunnel: [w125 w129] -> w109
          tunnel: [FALSE ("M4X Connected?") w128] -> w108
          frame False {
          }
          frame True {
            n55 = call "FT10_Connect M4X.vi"("error in (no error)"=w130, "reset device"=TRUE, "Board #"=u32 0, "Message Handling Cluster in"=w132) -> ("error out"=w129:errorcluster, "M4X Connected?"=w128:bool, "Message Handling Cluster out"=w131:T79)  [unwired: 4 in, 1 out]
          }
        }
        n56 = Bundle By Name(cluster=T75 {"Message"="", "Message Data"=variant} ("Message Cluster"), "Message Data"=w113, "Message"="Update Display") -> (w122:T75)
        n57 = Enqueue Element(queue=w119, element=w122, error in (no error)=w110) -> (error out=w121:errorcluster)  [unwired: 1 in, 2 out]
        n58 = Unbundle By Name(w111) -> ("M4X Connected?"=w118:refnum<vi>)
        n59 = property class="Bool (strict)"(reference=w118, "Value"=w108) -> ()  [unwired: 1 in, 2 out]
        n60 = Merge Errors(w109, w121) -> (w120:errorcluster)
      }
      frame "Unitherm Connect/Disconnect" {
        # "Connect or disconnect from Unitherm."
        n61 = Variant To Data(type=T96 {"Unitherm Connect/Disconnect"=FALSE, "Unitherm Refnum in"=""}, Variant=w138) -> (data=w145:T96)  [unwired: 1 in, 1 out]
        n62 = Unbundle By Name(w145) -> ("Unitherm Connect/Disconnect"=w136:T31)
        n63 = call "FT10_Connect Unitherm Handler.vi"("error in (no error)"=w139, "Message Data"=w138, "Message Handling Cluster in"=w143) -> ("error out"=w140:errorcluster, "Unitherm Connected?"=w141:bool, "Message Handling Cluster out"=w142:T79)  [unwired: 6 in]
        n64 = case shown="False" w136 {
          tunnel: ["Unitherm Disconnect" ("L10n_Action 1 Pressed") "Unitherm Connect" ("L10n_Action 1 Pressed")] -> w144
          frame False {
          }
          frame True {
          }
        }
        n65 = Unbundle By Name(w142) -> ("Unitherm Connected?"=w147:refnum<vi>)
        n66 = Bundle By Name(cluster=T75 {"Message"="", "Message Data"=variant} ("Message Cluster"), "Message Data"=w144, "Message"="Update Display") -> (w151:T75)
        n67 = Enqueue Element(queue=w148, element=w151, error in (no error)=w139) -> (error out=w150:errorcluster)  [unwired: 1 in, 2 out]
        n68 = property class="Bool (strict)"(reference=w147, "Value"=w141) -> ()  [unwired: 1 in, 2 out]
        n69 = Merge Errors(w140, w150) -> (w149:errorcluster)
      }
      frame "7854 Connect/Disconnect" {
        # "Connect or disconnect from Unitherm."
        n70 = Variant To Data(type=T97 {"PXI-7854R Resource"="PXI1Slot6", "75kHz"=TRUE, "uSec Off"=6, "uSec On"=7, "7854 Connect/Disconnect"=FALSE}, Variant=w159) -> (data=w164:T97)  [unwired: 1 in, 1 out]
        n71 = Unbundle By Name(w164) -> ("7854 Connect/Disconnect"=w162:T36)
        n72 = case shown="False" w162 {
          tunnel: ["PXI-7854R Disconnected" ("L10n_Action 1 Pressed") "PXI-7854R Connected" ("L10n_Action 1 Pressed")] -> w163
          frame False {
          }
          frame True {
          }
        }
        n73 = call "FT10_Connect FPGA_7854R Handler.vi"("error in"=w158, "Message Data"=w159, "Message Handling Cluster in"=w161) -> ("error out"=w157:errorcluster, "PXI-7854R Connected?"=w156:bool, "Message Handling Cluster out"=w160:T79)  [unwired: 6 in]
        n74 = Unbundle By Name(w160) -> ("PXI-7854R Connected?"=w166:refnum<vi>)
        n75 = Bundle By Name(cluster=T75 {"Message"="", "Message Data"=variant} ("Message Cluster"), "Message Data"=w163, "Message"="Update Display") -> (w170:T75)
        n76 = Enqueue Element(queue=w167, element=w170, error in (no error)=w158) -> (error out=w169:errorcluster)  [unwired: 1 in, 2 out]
        n77 = property class="Bool (strict)"(reference=w166, "Value"=w156) -> ()  [unwired: 1 in, 2 out]
        n78 = Merge Errors(w157, w169) -> (w168:errorcluster)
      }
      frame "Set Load" {
        # "Adjust the Impedance of the Unitherm."
        n79 = Variant To Data(type=0 ("Load (Ohms)"), Variant=w186) -> (data=w178:i32)  [unwired: 1 in, 1 out]
        n80 = Number To Decimal String(number=w178) -> (decimal integer string=w180:string)  [unwired: 1 in]
        n81 = Unbundle By Name(w189) -> ("UNITHERM Connection"=w185:refnum<visa-resource-name>)
        n82 = Concatenate Strings("Unitherm Load set to " ("L10n_Action 1 Pressed"), w180, " Ohms" ("string")) -> (w181:string)
        n83 = call "FT10_Unitherm Set Load.vi"("error in (no error)"=w182, "Load Impedance in"=w178, "VISA Refnum in"=w185) -> ("error out"=w183:errorcluster, "Load Impedance out"=w175:i32, "VISA Refnum out"=w184:refnum<visa-resource-name>, "Set Load Case"=→"Set Load Case":string)  [unwired: 5 in]
        n84 = Bundle By Name(cluster=T75 {"Message"="", "Message Data"=variant} ("Message Cluster"), "Message"="Update Display", "Message Data"=w181) -> (w191:T75)
        n85 = Bundle By Name(cluster=w189, "UNITHERM Connection"=w184) -> (w177:T79)
        n86 = Enqueue Element(queue=w195, element=w191, error in (no error)=w182) -> (error out=w194:errorcluster)  [unwired: 1 in, 2 out]
        n87 = Merge Errors(w183, w194) -> (w188:errorcluster)
        n88 = call "FT10_Log Update Unitherm Load Value.vi"("Load Impedance in"=w175, "Message Handling Cluster in"=w177) -> ("Message Handling Cluster out"=w176:T79)  [unwired: 9 in]
      }
      frame "Clear Load" {
        # "Adjust the Impedance of the Unitherm."
        n89 = Unbundle By Name(w205) -> ("UNITHERM Connection"=w202:refnum<visa-resource-name>)
        n90 = call "FT10_Unitherm Clear Load.vi"("error in (no error)"=w200, "VISA Refnum in"=w202) -> ("error out"=w199:errorcluster, "Load Impedance out"=w196:i32, "VISA Refnum out"=w201:refnum<visa-resource-name>)  [unwired: 7 in]
        n91 = Bundle By Name(cluster=T75 {"Message"="", "Message Data"=variant} ("Message Cluster"), "Message"="Update Display", "Message Data"="Unitherm Load Cleared" ("L10n_Action 1 Pressed")) -> (w206:T75)
        n92 = Bundle By Name(cluster=w205, "UNITHERM Connection"=w201) -> (w198:T79)
        n93 = Enqueue Element(queue=w210, element=w206, error in (no error)=w200) -> (error out=w209:errorcluster)  [unwired: 1 in, 2 out]
        n94 = Merge Errors(w199, w209) -> (w204:errorcluster)
        n95 = call "FT10_Log Update Unitherm Load Value.vi"("Load Impedance in"=w196, "Message Handling Cluster in"=w198) -> ("Message Handling Cluster out"=w197:T79)  [unwired: 9 in]
      }
      frame "Read Current" {
        # "Read data from M4X and send to logging loop if logging is enabled."
        n96 = global read "Abort Auto Test Global.vi" "Abort Auto Test"() -> (w211:bool)
        n97 = case shown="False" w211 {
          tunnel: w217 -> [w226 w227]
          tunnel: [w223 w227] -> w213
          frame False {
            n98 = call "FT10_M4X Read.vi"("Message Handling Cluster in"=w226) -> ("Waveform Array"=→"Data":waveform(dbl)[], "Analysis Cluster Array"=→"Array":T1, "Message Handling Cluster out"=w223:T79)  [unwired: 8 in]
          }
          frame True {
          }
        }
        n99 = Bundle By Name(cluster=T75 {"Message"="", "Message Data"=variant} ("Message Cluster"), "Message"="Update Display", "Message Data"="\"Read Current\" pressed" ("L10n_Action 1 Pressed")) -> (w218:T75)
        n100 = call "FT10_Log Queue Data.vi"("Message Handling Cluster in"=w213) -> ("Message Handling Cluster out"=w212:T79)  [unwired: 10 in]
        n101 = Enqueue Element(queue=w222, element=w218, error in (no error)=w214) -> (error out=w221:errorcluster)  [unwired: 1 in, 2 out]
        n102 = Merge Errors(w221) -> (w216:errorcluster)
      }
      frame "7854 Set Config" {
        n103 = global read "Abort Auto Test Global.vi" "Abort Auto Test"() -> (w229:bool)
        n104 = Variant To Data(type=T98 {"7854 Config Enum"=enum."Mono 1", "7854 Set Config"=FALSE}, Variant=w239) -> (data=w242:T98)  [unwired: 1 in, 1 out]
        n105 = Unbundle By Name(w242) -> ("7854 Config Enum"=w228:T42)
        n106 = case shown="False" w229 {
          tunnel: w241 -> [w249 w259]
          tunnel: [w248 w258] -> w240
          tunnel: w228 -> [w244 _]
          frame False {
            n107 = Unbundle By Name(w249) -> ("FPGA VI Reference Out"=w247:T81)
            n108 = case shown="\"BiPolar\"" w244 {
              tunnel: [T99."Off" ("Update Config Enum") T99."Mono1 Relay Config" ("Update Config Enum") T99."Mono2 Relay Config" ("Update Config Enum") T99."Bipolar Relay Config" ("Update Config Enum") T99."Ligasure Relay Config" ("Update Config Enum")] -> w245
              frame "Off" {
              }
              frame "Mono 1" {
              }
              frame "Mono 2" {
              }
              frame "BiPolar" {
              }
              frame "LigaSure" {
              }
            }
            n109 = call "FT10_FPGA_7854R Set Relay Config.vi"("Update Config Enum"=w245, "Refnum in"=w247) -> ("Refnum out"=w246:T81)  [unwired: 9 in]
            n110 = Bundle By Name(cluster=w249, "FPGA VI Reference Out"=w246) -> (w248:T79)
          }
          frame True {
            n111 = Unbundle By Name(w259) -> ("FPGA VI Reference Out"=w256:T81)
            n112 = call "FT10_FPGA_7854R Set Relay Config.vi"("Update Config Enum"=T99."Off", "Refnum in"=w256) -> ("Refnum out"=w257:T81)  [unwired: 9 in]
            n113 = Bundle By Name(cluster=w259, "FPGA VI Reference Out"=w257) -> (w258:T79)
          }
        }
        n114 = call "FT10_FPGA_7854R Set Config.vi"("7854 Config Enum"=w228) -> ("Config string"=w232:string)  [unwired: 7 in, 3 out]
        n115 = Concatenate Strings("PXI-7854R Configuration Set to " ("Display Message"), w232) -> (w231:string)
        n116 = Bundle By Name(cluster=T75 {"Message"="", "Message Data"=variant} ("Message Cluster"), "Message"="Update Display", "Message Data"=w231) -> (w235:T75)
        n117 = Enqueue Element(queue=w230, element=w235, error in (no error)=w233) -> (error out=w234:errorcluster)  [unwired: 1 in, 2 out]
      }
      frame "Auto Set Power" {
        n118 = Variant To Data(type=T100 {"Port"=enum."Mono1", "Mode"=enum."Pure", "Power Level"=0.0}, Variant=w273) -> (data=w263:T100)  [unwired: 1 in, 1 out]
        n119 = global read "Abort Auto Test Global.vi" "Abort Auto Test"() -> (w260:bool)
        n120 = case shown="False" w260 {
          tunnel: w264 -> [w276 w277]
          tunnel: w263 -> [w275 _]
          tunnel: [w274 w277] -> w261
          frame False {
            n121 = call "FT10_Semi-Auto Power Set and Read.vi"("Auto Set Power Cluster in"=w275, "Message Handling Cluster in"=w276) -> ("Message Handling Cluster out"=w274:T79)  [unwired: 8 in, 1 out]
          }
          frame True {
          }
        }
        n122 = call "FT10_Semi-Auto Set Power Display String.vi"("Auto Set Power Cluster"=w263) -> ("Display String"=w265:string)  [unwired: 10 in]
        n123 = Bundle By Name(cluster=T75 {"Message"="", "Message Data"=variant} ("Message Cluster"), "Message"="Update Display", "Message Data"=w265) -> (w270:T75)
        n124 = call "FT10_Fornax Read and Parse.vi"("Message Handling Cluster in"=w261) -> ("Message Handling Cluster out"=w262:T79)  [unwired: 9 in, 1 out]
        n125 = Enqueue Element(queue=w267, element=w270, error in (no error)=w268) -> (error out=w269:errorcluster)  [unwired: 1 in, 2 out]
      }
      frame "Mono1 Cut Activate Port" {
        # "Turn power ON or OFF on MONO1 Cut Port"
        n126 = Variant To Data(type=T14 FALSE ("Mono1 Cut Activate"), Variant=w283) -> (data=w278:T14)  [unwired: 1 in, 1 out]
        n127 = Unbundle By Name(w285) -> ("Fornax Connection"=w282:refnum<k5>)
        n128 = call "FT10_Fornax Mono1 Cut Activate Port Command.vi"("Mono1 Cut Activate"=w278, "TCP Network Connection in"=w282) -> ("TCP Network Connection out"=w281:refnum<k5>)  [unwired: 9 in]
        n129 = Bundle By Name(cluster=w285, "Fornax Connection"=w281) -> (w280:T79)
        n130 = Bundle By Name(cluster=T75 {"Message"="", "Message Data"=variant} ("Message Cluster"), "Message"="Update Display", "Message Data"="\"Mono1 Cut Activate Port\" pressed" ("L10n_Action 1 Pressed")) -> (w290:T75)
        n131 = call "FT10_Log Update Mono1 Cut Log.vi"("Mono1 Cut Activate"=w278, "Message Handling Cluster in"=w280) -> ("Message Handling Cluster out"=w279:T79)  [unwired: 9 in]
        n132 = Enqueue Element(queue=w288, element=w290, error in (no error)=w287) -> (error out=w286:errorcluster)  [unwired: 1 in, 2 out]
      }
      frame "Mono2 Cut Activate Port" {
        # "Turn power ON or OFF on MONO2 Cut Port"
        n133 = Variant To Data(type=T22 FALSE ("Mono2 Cut Activate"), Variant=w299) -> (data=w293:T22)  [unwired: 1 in, 1 out]
        n134 = Unbundle By Name(w300) -> ("Fornax Connection"=w297:refnum<k5>)
        n135 = call "FT10_Fornax Mono2 Cut Activate Port Command.vi"("Mono2 Cut Activate"=w293, "TCP Network Connection in"=w297) -> ("TCP Network Connection out"=w296:refnum<k5>)  [unwired: 9 in]
        n136 = Bundle By Name(cluster=w300, "Fornax Connection"=w296) -> (w295:T79)
        n137 = Bundle By Name(cluster=T75 {"Message"="", "Message Data"=variant} ("Message Cluster"), "Message"="Update Display", "Message Data"="\"Mono2 Cut Activate Port\" pressed" ("L10n_Action 1 Pressed")) -> (w305:T75)
        n138 = call "FT10_Log Update Mono2 Cut Log.vi"("Mono2 Cut Activate"=w293, "Message Handling Cluster in"=w295) -> ("Message Handling Cluster out"=w294:T79)  [unwired: 9 in]
        n139 = Enqueue Element(queue=w303, element=w305, error in (no error)=w302) -> (error out=w301:errorcluster)  [unwired: 1 in, 2 out]
      }
      frame "Mono1 Coag Activate Port" {
        # "Turn power ON or OFF on MONO1 Coag Port"
        n140 = Variant To Data(type=T19 FALSE ("Mono1 Coag Activate"), Variant=w314) -> (data=w308:T19)  [unwired: 1 in, 1 out]
        n141 = Unbundle By Name(w315) -> ("Fornax Connection"=w312:refnum<k5>)
        n142 = call "FT10_Fornax Mono1 Coag Activate Port Command.vi"("Mono1 Coag Activate"=w308, "TCP Network Connection in"=w312) -> ("TCP Network Connection out"=w311:refnum<k5>)  [unwired: 9 in]
        n143 = Bundle By Name(cluster=w315, "Fornax Connection"=w311) -> (w310:T79)
        n144 = Bundle By Name(cluster=T75 {"Message"="", "Message Data"=variant} ("Message Cluster"), "Message"="Update Display", "Message Data"="\"Mono1 Coag Activate Port\" pressed" ("L10n_Action 1 Pressed")) -> (w320:T75)
        n145 = call "FT10_Log Update Mono1 Coag Log.vi"("Mono1 Coag Activate"=w308, "Message Handling Cluster in"=w310) -> ("Message Handling Cluster out"=w309:T79)  [unwired: 9 in]
        n146 = Enqueue Element(queue=w318, element=w320, error in (no error)=w317) -> (error out=w316:errorcluster)  [unwired: 1 in, 2 out]
      }
      frame "Mono2 Coag Activate Port" {
        # "Turn power ON or OFF on MONO2 Coag Port"
        n147 = Variant To Data(type=T26 FALSE ("Mono2 Coag Activate"), Variant=w328) -> (data=w323:T26)  [unwired: 1 in, 1 out]
        n148 = Unbundle By Name(w330) -> ("Fornax Connection"=w327:refnum<k5>)
        n149 = call "FT10_Fornax Mono2 Coag Activate Port Command.vi"("Mono2 Coag Activate"=w323, "TCP Network Connection in"=w327) -> ("TCP Network Connection out"=w326:refnum<k5>)  [unwired: 9 in]
        n150 = Bundle By Name(cluster=w330, "Fornax Connection"=w326) -> (w325:T79)
        n151 = Bundle By Name(cluster=T75 {"Message"="", "Message Data"=variant} ("Message Cluster"), "Message"="Update Display", "Message Data"="\"Mono2 Coag Activate Port\" pressed" ("L10n_Action 1 Pressed")) -> (w335:T75)
        n152 = call "FT10_Log Update Mono2 Coag Log.vi"("Mono2 Coag Activate"=w323, "Message Handling Cluster in"=w325) -> ("Message Handling Cluster out"=w324:T79)  [unwired: 9 in]
        n153 = Enqueue Element(queue=w333, element=w335, error in (no error)=w332) -> (error out=w331:errorcluster)  [unwired: 1 in, 2 out]
      }
      frame "Ligasure Activate Port" {
        # "Turn power ON or OFF on Ligasure Port"
        n154 = Variant To Data(type=T9 FALSE ("Ligasure Activate"), Variant=w343) -> (data=w338:T9)  [unwired: 1 in, 1 out]
        n155 = Unbundle By Name(w345) -> ("Fornax Connection"=w342:refnum<k5>)
        n156 = call "FT10_Fornax Ligasure Activate Port Command.vi"("Ligasure Activate"=w338, "TCP Network Connection in"=w342) -> ("TCP Network Connection out"=w341:refnum<k5>)  [unwired: 9 in]
        n157 = Bundle By Name(cluster=w345, "Fornax Connection"=w341) -> (w340:T79)
        n158 = Bundle By Name(cluster=T75 {"Message"="", "Message Data"=variant} ("Message Cluster"), "Message"="Update Display", "Message Data"="\"Ligasure Activate Port\" pressed" ("L10n_Action 1 Pressed")) -> (w350:T75)
        n159 = call "FT10_Log Update Ligasure Log.vi"("Ligasure Activate"=w338, "Message Handling Cluster in"=w340) -> ("Message Handling Cluster out"=w339:T79)  [unwired: 9 in]
        n160 = Enqueue Element(queue=w348, element=w350, error in (no error)=w347) -> (error out=w346:errorcluster)  [unwired: 1 in, 2 out]
      }
      frame "Bipolar Activate Port" {
        # "Turn power ON or OFF on Bipolar Port"
        n161 = Variant To Data(type=T10 FALSE ("Bipolar Activate"), Variant=w358) -> (data=w353:T10)  [unwired: 1 in, 1 out]
        n162 = Unbundle By Name(w360) -> ("Fornax Connection"=w357:refnum<k5>)
        n163 = call "FT10_Fornax Bipolar Activate Port Command.vi"("Bipolar Activate"=w353, "TCP Network Connection in"=w357) -> ("TCP Network Connection out"=w356:refnum<k5>)  [unwired: 9 in]
        n164 = Bundle By Name(cluster=w360, "Fornax Connection"=w356) -> (w355:T79)
        n165 = Bundle By Name(cluster=T75 {"Message"="", "Message Data"=variant} ("Message Cluster"), "Message"="Update Display", "Message Data"="\"Bipolar Activate Port\" pressed" ("L10n_Action 1 Pressed")) -> (w365:T75)
        n166 = call "FT10_Log Update Bipolar Log.vi"("Bipolar Activate"=w353, "Message Handling Cluster in"=w355) -> ("Message Handling Cluster out"=w354:T79)  [unwired: 9 in]
        n167 = Enqueue Element(queue=w363, element=w365, error in (no error)=w362) -> (error out=w361:errorcluster)  [unwired: 1 in, 2 out]
      }
      frame "Mono1 Cut - Handswitch Activate Port" {
        n168 = Variant To Data(type=TRUE, Variant=w380) -> (data=w371:bool)  [unwired: 1 in, 1 out]
        n169 = case shown="False" w371 {
          tunnel: [T99."Handswitch - Mono1 Cut" ("Update Config Enum") T99."Mono1 Relay Config" ("Update Config Enum")] -> w368
          frame True {
          }
          frame False {
          }
        }
        n170 = Unbundle By Name(w382) -> ("FPGA VI Reference Out"=w370:T81)
        n171 = call "FT10_FPGA_7854R Set Relay Config.vi"("Update Config Enum"=w368, "Refnum in"=w370) -> ("Refnum out"=w369:T81)  [unwired: 9 in]
        n172 = Bundle By Name(cluster=T75 {"Message"="", "Message Data"=variant} ("Message Cluster"), "Message"="Update Display", "Message Data"="Mono1 Cut - Handswitch Activate Port" ("Display Message")) -> (w377:T75)
        n173 = Bundle By Name(cluster=w382, "FPGA VI Reference Out"=w369) -> (w381:T79)
        n174 = Enqueue Element(queue=w373, element=w377, error in (no error)=w375) -> (error out=w376:errorcluster)  [unwired: 1 in, 2 out]
      }
      frame "Mono1 Coag - Handswitch Activate Port" {
        n175 = Variant To Data(type=TRUE, Variant=w397) -> (data=w388:bool)  [unwired: 1 in, 1 out]
        n176 = case shown="True" w388 {
          tunnel: [T99."Handswitch - Mono1 Coag" ("Update Config Enum") T99."Mono1 Relay Config" ("Update Config Enum")] -> w385
          frame True {
          }
          frame False {
          }
        }
        n177 = Unbundle By Name(w399) -> ("FPGA VI Reference Out"=w387:T81)
        n178 = call "FT10_FPGA_7854R Set Relay Config.vi"("Update Config Enum"=w385, "Refnum in"=w387) -> ("Refnum out"=w386:T81)  [unwired: 9 in]
        n179 = Bundle By Name(cluster=T75 {"Message"="", "Message Data"=variant} ("Message Cluster"), "Message"="Update Display", "Message Data"="Mono1 Coag - Handswitch Activate Port" ("Display Message")) -> (w394:T75)
        n180 = Bundle By Name(cluster=w399, "FPGA VI Reference Out"=w386) -> (w398:T79)
        n181 = Enqueue Element(queue=w390, element=w394, error in (no error)=w392) -> (error out=w393:errorcluster)  [unwired: 1 in, 2 out]
      }
      frame "Mono2 Cut - Handswitch Activate Port" {
        n182 = Variant To Data(type=TRUE, Variant=w414) -> (data=w405:bool)  [unwired: 1 in, 1 out]
        n183 = case shown="False" w405 {
          tunnel: [T99."Handswitch - Mono2 Cut" ("Update Config Enum") T99."Mono2 Relay Config" ("Update Config Enum")] -> w402
          frame True {
          }
          frame False {
          }
        }
        n184 = Unbundle By Name(w416) -> ("FPGA VI Reference Out"=w403:T81)
        n185 = call "FT10_FPGA_7854R Set Relay Config.vi"("Update Config Enum"=w402, "Refnum in"=w403) -> ("Refnum out"=w404:T81)  [unwired: 9 in]
        n186 = Bundle By Name(cluster=T75 {"Message"="", "Message Data"=variant} ("Message Cluster"), "Message"="Update Display", "Message Data"="Mono2 Cut - Handswitch Activate Port" ("Display Message")) -> (w411:T75)
        n187 = Bundle By Name(cluster=w416, "FPGA VI Reference Out"=w404) -> (w415:T79)
        n188 = Enqueue Element(queue=w407, element=w411, error in (no error)=w409) -> (error out=w410:errorcluster)  [unwired: 1 in, 2 out]
      }
      frame "Mono2 Coag - Handswitch Activate Port" {
        n189 = Variant To Data(type=TRUE, Variant=w431) -> (data=w422:bool)  [unwired: 1 in, 1 out]
        n190 = case shown="True" w422 {
          tunnel: [T99."Handswitch - Mono2 Coag" ("Update Config Enum") T99."Mono2 Relay Config" ("Update Config Enum")] -> w419
          frame True {
          }
          frame False {
          }
        }
        n191 = Unbundle By Name(w433) -> ("FPGA VI Reference Out"=w420:T81)
        n192 = call "FT10_FPGA_7854R Set Relay Config.vi"("Update Config Enum"=w419, "Refnum in"=w420) -> ("Refnum out"=w421:T81)  [unwired: 9 in]
        n193 = Bundle By Name(cluster=T75 {"Message"="", "Message Data"=variant} ("Message Cluster"), "Message"="Update Display", "Message Data"="Mono2 Coag - Handswitch Activate Port" ("Display Message")) -> (w428:T75)
        n194 = Bundle By Name(cluster=w433, "FPGA VI Reference Out"=w421) -> (w432:T79)
        n195 = Enqueue Element(queue=w424, element=w428, error in (no error)=w426) -> (error out=w427:errorcluster)  [unwired: 1 in, 2 out]
      }
      frame "Mono2 Triverse Tab" {
        n196 = Variant To Data(type=enum32{"Mono 2 - 2 Button", "Mono 2 - Triverse"}."Mono 2 - Triverse" ("Mono2 Triverse Tab"), Variant=w448) -> (data=w440:enum32{"Mono 2 - 2 Button", "Mono 2 - Triverse"})  [unwired: 1 in, 1 out]
        n197 = case shown="\"Mono 2 - Triverse\"" w440 {
          tunnel: [T99."Switch to Triverse Mode" ("Update Config Enum") T99."Switch to Mono2 - 2 button Mode" ("Update Config Enum")] -> w436
          frame "Mono 2 - Triverse" {
          }
          frame "Mono 2 - 2 Button", Default {
          }
        }
        n198 = Unbundle By Name(w450) -> ("FPGA VI Reference Out"=w437:T81)
        n199 = call "FT10_FPGA_7854R Set Relay Config.vi"("Update Config Enum"=w436, "Refnum in"=w437) -> ("Refnum out"=w438:T81)  [unwired: 9 in]
        n200 = Bundle By Name(cluster=T75 {"Message"="", "Message Data"=variant} ("Message Cluster"), "Message"="Update Display", "Message Data"="Mono2 Tab switched" ("Display Message")) -> (w445:T75)
        n201 = Bundle By Name(cluster=w450, "FPGA VI Reference Out"=w438) -> (w449:T79)
        n202 = Enqueue Element(queue=w441, element=w445, error in (no error)=w443) -> (error out=w444:errorcluster)  [unwired: 1 in, 2 out]
      }
      frame "Triverse Slide" {
        n203 = Variant To Data(type=i8 1 ("Triverse Slide"), Variant=w465) -> (data=w457:i8)  [unwired: 1 in, 1 out]
        n204 = case shown="5" w457 {
          tunnel: [T99."Triverse Power 1" ("Update Config Enum") T99."Triverse Power 2" ("Update Config Enum") T99."Triverse Power 3" ("Update Config Enum") T99."Triverse Power 4" ("Update Config Enum") T99."Triverse Power 5" ("Update Config Enum")] -> w453
          frame 1, Default {
          }
          frame 2 {
          }
          frame 3 {
          }
          frame 4 {
          }
          frame 5 {
          }
        }
        n205 = Unbundle By Name(w467) -> ("FPGA VI Reference Out"=w454:T81)
        n206 = call "FT10_FPGA_7854R Set Relay Config.vi"("Update Config Enum"=w453, "Refnum in"=w454) -> ("Refnum out"=w455:T81)  [unwired: 9 in]
        n207 = Bundle By Name(cluster=T75 {"Message"="", "Message Data"=variant} ("Message Cluster"), "Message"="Update Display", "Message Data"="Triverse Slide updated" ("Display Message")) -> (w462:T75)
        n208 = Bundle By Name(cluster=w467, "FPGA VI Reference Out"=w455) -> (w466:T79)
        n209 = Enqueue Element(queue=w458, element=w462, error in (no error)=w460) -> (error out=w461:errorcluster)  [unwired: 1 in, 2 out]
      }
      frame "Mono2 Triverse - Handswitch Seal" {
        n210 = Variant To Data(type=FALSE ("Mono2 Triverse - Handswitch Seal"), Variant=w485) -> (data=w477:bool)  [unwired: 1 in, 1 out]
        n211 = case shown="True" w477 {
          tunnel: [T99."Mono2 Relay Config" ("Update Config Enum") T99."Handswitch - Triverse Seal" ("Update Config Enum")] -> w473
          frame False {
          }
          frame True {
          }
        }
        n212 = Unbundle By Name(w487) -> ("FPGA VI Reference Out"=w474:T81)
        n213 = call "FT10_FPGA_7854R Set Relay Config.vi"("Update Config Enum"=w473, "Refnum in"=w474) -> ("Refnum out"=w475:T81)  [unwired: 9 in]
        n214 = Bundle By Name(cluster=T75 {"Message"="", "Message Data"=variant} ("Message Cluster"), "Message"="Update Display", "Message Data"="Mono2 Triverse - Handswitch Seal updated" ("Display Message")) -> (w482:T75)
        n215 = Bundle By Name(cluster=w487, "FPGA VI Reference Out"=w475) -> (w486:T79)
        n216 = Enqueue Element(queue=w478, element=w482, error in (no error)=w480) -> (error out=w481:errorcluster)  [unwired: 1 in, 2 out]
      }
      frame "Mono2 Triverse - Handswitch Cut" {
        n217 = Variant To Data(type=FALSE ("Mono2 Triverse - Handswitch Seal"), Variant=w502) -> (data=w494:bool)  [unwired: 1 in, 1 out]
        n218 = case shown="False" w494 {
          tunnel: [T99."Mono2 Relay Config" ("Update Config Enum") T99."Handswitch - Triverse Cut" ("Update Config Enum")] -> w490
          frame False {
          }
          frame True {
          }
        }
        n219 = Unbundle By Name(w504) -> ("FPGA VI Reference Out"=w492:T81)
        n220 = call "FT10_FPGA_7854R Set Relay Config.vi"("Update Config Enum"=w490, "Refnum in"=w492) -> ("Refnum out"=w491:T81)  [unwired: 9 in]
        n221 = Bundle By Name(cluster=T75 {"Message"="", "Message Data"=variant} ("Message Cluster"), "Message"="Update Display", "Message Data"="Mono2 Triverse - Handswitch Cut updated" ("Display Message")) -> (w499:T75)
        n222 = Bundle By Name(cluster=w504, "FPGA VI Reference Out"=w491) -> (w503:T79)
        n223 = Enqueue Element(queue=w495, element=w499, error in (no error)=w497) -> (error out=w498:errorcluster)  [unwired: 1 in, 2 out]
      }
      frame "Mono2 Triverse - Handswitch Coag" {
        n224 = Variant To Data(type=FALSE ("Mono2 Triverse - Handswitch Seal"), Variant=w519) -> (data=w511:bool)  [unwired: 1 in, 1 out]
        n225 = case shown="True" w511 {
          tunnel: [T99."Mono2 Relay Config" ("Update Config Enum") T99."Handswitch - Triverse Coag" ("Update Config Enum")] -> w507
          frame False {
          }
          frame True {
          }
        }
        n226 = Unbundle By Name(w521) -> ("FPGA VI Reference Out"=w508:T81)
        n227 = call "FT10_FPGA_7854R Set Relay Config.vi"("Update Config Enum"=w507, "Refnum in"=w508) -> ("Refnum out"=w509:T81)  [unwired: 9 in]
        n228 = Bundle By Name(cluster=T75 {"Message"="", "Message Data"=variant} ("Message Cluster"), "Message"="Update Display", "Message Data"="Mono2 Triverse - Handswitch Coag updated" ("Display Message")) -> (w516:T75)
        n229 = Bundle By Name(cluster=w521, "FPGA VI Reference Out"=w509) -> (w520:T79)
        n230 = Enqueue Element(queue=w512, element=w516, error in (no error)=w514) -> (error out=w515:errorcluster)  [unwired: 1 in, 2 out]
      }
      frame "Mono1 Cut - Footswitch Activate Port" {
        n231 = Bundle By Name(cluster=w536, "Footswitch Cluster.PXI-2565 resource name"=w535) -> (w534:T79)
        n232 = Variant To Data(type=TRUE, Variant=w544) -> (data=w528:bool)  [unwired: 1 in, 1 out]
        n233 = call "FT10_PXI-2565 Connect.vi"("error in (no error)"=w533, "Message Handling Cluster in"=w534) -> ("error out"=w529:errorcluster, "Message Handling Cluster out"=w531:T79)  [unwired: 8 in]
        n234 = call "FT10_PXI-2565 Switch Relay.vi"("Activate?"=w528, "error in (no error)"=w529, "Channel 2"="com1" ("channel 2"), "Channel 1"="ch1" ("channel 1"), "Message Handling Cluster in"=w531) -> ("error out"=w525:errorcluster, "Connected?"=w524:bool, "Message Handling Cluster out"=w530:T79)  [unwired: 4 in]
        n235 = local write "Connected?"(w524) -> ()
        n236 = Merge Errors(w525, w533) -> (w532:errorcluster)
        n237 = Bundle By Name(cluster=T75 {"Message"="", "Message Data"=variant} ("Message Cluster"), "Message"="Update Display", "Message Data"="Mono1 Cut - Footswitch Activate Port" ("Display Message")) -> (w541:T75)
        n238 = Enqueue Element(queue=w538, element=w541, error in (no error)=w532) -> (error out=w540:errorcluster)  [unwired: 1 in, 2 out]
      }
      frame "Mono1 Coag - Footswitch Activate Port" {
        n239 = Bundle By Name(cluster=w557, "Footswitch Cluster.PXI-2565 resource name"=w556) -> (w555:T79)
        n240 = Variant To Data(type=TRUE, Variant=w565) -> (data=w549:bool)  [unwired: 1 in, 1 out]
        n241 = call "FT10_PXI-2565 Connect.vi"("error in (no error)"=w554, "Message Handling Cluster in"=w555) -> ("error out"=w550:errorcluster, "Message Handling Cluster out"=w552:T79)  [unwired: 8 in]
        n242 = call "FT10_PXI-2565 Switch Relay.vi"("Activate?"=w549, "error in (no error)"=w550, "Channel 2"="com0" ("channel 2"), "Channel 1"="ch0" ("channel 1"), "Message Handling Cluster in"=w552) -> ("error out"=w546:errorcluster, "Connected?"=w545:bool, "Message Handling Cluster out"=w551:T79)  [unwired: 4 in]
        n243 = local write "Connected?"(w545) -> ()
        n244 = Merge Errors(w546, w554) -> (w553:errorcluster)
        n245 = Bundle By Name(cluster=T75 {"Message"="", "Message Data"=variant} ("Message Cluster"), "Message"="Update Display", "Message Data"="Mono1 Coag - Footswitch Activate Port" ("Display Message")) -> (w562:T75)
        n246 = Enqueue Element(queue=w559, element=w562, error in (no error)=w553) -> (error out=w561:errorcluster)  [unwired: 1 in, 2 out]
      }
      frame "Mono2 Cut - Footswitch Activate Port" {
        n247 = Bundle By Name(cluster=w578, "Footswitch Cluster.PXI-2565 resource name"=w577) -> (w576:T79)
        n248 = Variant To Data(type=TRUE, Variant=w586) -> (data=w570:bool)  [unwired: 1 in, 1 out]
        n249 = call "FT10_PXI-2565 Connect.vi"("error in (no error)"=w575, "Message Handling Cluster in"=w576) -> ("error out"=w571:errorcluster, "Message Handling Cluster out"=w573:T79)  [unwired: 8 in]
        n250 = call "FT10_PXI-2565 Switch Relay.vi"("Activate?"=w570, "error in (no error)"=w571, "Channel 2"="com4" ("channel 2"), "Channel 1"="ch4" ("channel 1"), "Message Handling Cluster in"=w573) -> ("error out"=w567:errorcluster, "Connected?"=→"Connected?":bool, "Message Handling Cluster out"=w572:T79)  [unwired: 4 in]
        n251 = Merge Errors(w567, w575) -> (w574:errorcluster)
        n252 = Bundle By Name(cluster=T75 {"Message"="", "Message Data"=variant} ("Message Cluster"), "Message"="Update Display", "Message Data"="Mono2 Cut - Footswitch Activate Port" ("Display Message")) -> (w583:T75)
        n253 = Enqueue Element(queue=w580, element=w583, error in (no error)=w574) -> (error out=w582:errorcluster)  [unwired: 1 in, 2 out]
      }
      frame "Mono2 Coag - Footswitch Activate Port" {
        n254 = Bundle By Name(cluster=w599, "Footswitch Cluster.PXI-2565 resource name"=w598) -> (w597:T79)
        n255 = Variant To Data(type=TRUE, Variant=w607) -> (data=w591:bool)  [unwired: 1 in, 1 out]
        n256 = call "FT10_PXI-2565 Connect.vi"("error in (no error)"=w596, "Message Handling Cluster in"=w597) -> ("error out"=w592:errorcluster, "Message Handling Cluster out"=w594:T79)  [unwired: 8 in]
        n257 = call "FT10_PXI-2565 Switch Relay.vi"("Activate?"=w591, "error in (no error)"=w592, "Channel 2"="com3" ("channel 2"), "Channel 1"="ch3" ("channel 1"), "Message Handling Cluster in"=w594) -> ("error out"=w588:errorcluster, "Connected?"=w587:bool, "Message Handling Cluster out"=w593:T79)  [unwired: 4 in]
        n258 = local write "Connected?"(w587) -> ()
        n259 = Merge Errors(w588, w596) -> (w595:errorcluster)
        n260 = Bundle By Name(cluster=T75 {"Message"="", "Message Data"=variant} ("Message Cluster"), "Message"="Update Display", "Message Data"="Mono2 Coag - Footswitch Activate Port" ("Display Message")) -> (w604:T75)
        n261 = Enqueue Element(queue=w601, element=w604, error in (no error)=w595) -> (error out=w603:errorcluster)  [unwired: 1 in, 2 out]
      }
      frame "Mono2 Triverse - Footswitch Activate Port" {
        n262 = Bundle By Name(cluster=w620, "Footswitch Cluster.PXI-2565 resource name"=w619) -> (w618:T79)
        n263 = Variant To Data(type=TRUE, Variant=w628) -> (data=w612:bool)  [unwired: 1 in, 1 out]
        n264 = call "FT10_PXI-2565 Connect.vi"("error in (no error)"=w617, "Message Handling Cluster in"=w618) -> ("error out"=w613:errorcluster, "Message Handling Cluster out"=w615:T79)  [unwired: 8 in]
        n265 = call "FT10_PXI-2565 Switch Relay.vi"("Activate?"=w612, "error in (no error)"=w613, "Channel 2"="com5" ("channel 2"), "Channel 1"="ch5" ("channel 1"), "Message Handling Cluster in"=w615) -> ("error out"=w609:errorcluster, "Connected?"=w608:bool, "Message Handling Cluster out"=w614:T79)  [unwired: 4 in]
        n266 = local write "Connected?"(w608) -> ()
        n267 = Merge Errors(w609, w617) -> (w616:errorcluster)
        n268 = Bundle By Name(cluster=T75 {"Message"="", "Message Data"=variant} ("Message Cluster"), "Message"="Update Display", "Message Data"="Mono2 Triverse - Footswitch Activate Port" ("Display Message")) -> (w625:T75)
        n269 = Enqueue Element(queue=w622, element=w625, error in (no error)=w616) -> (error out=w624:errorcluster)  [unwired: 1 in, 2 out]
      }
      frame "Bipolar - Footswitch Activate Port" {
        n270 = Bundle By Name(cluster=w641, "Footswitch Cluster.PXI-2565 resource name"=w640) -> (w639:T79)
        n271 = Variant To Data(type=TRUE, Variant=w649) -> (data=w633:bool)  [unwired: 1 in, 1 out]
        n272 = call "FT10_PXI-2565 Connect.vi"("error in (no error)"=w638, "Message Handling Cluster in"=w639) -> ("error out"=w634:errorcluster, "Message Handling Cluster out"=w636:T79)  [unwired: 8 in]
        n273 = call "FT10_PXI-2565 Switch Relay.vi"("Activate?"=w633, "error in (no error)"=w634, "Channel 2"="com8" ("channel 2"), "Channel 1"="ch8" ("channel 1"), "Message Handling Cluster in"=w636) -> ("error out"=w630:errorcluster, "Connected?"=w629:bool, "Message Handling Cluster out"=w635:T79)  [unwired: 4 in]
        n274 = local write "Connected?"(w629) -> ()
        n275 = Merge Errors(w630, w638) -> (w637:errorcluster)
        n276 = Bundle By Name(cluster=T75 {"Message"="", "Message Data"=variant} ("Message Cluster"), "Message"="Update Display", "Message Data"="Bipolar - Footswitch Activate Port" ("Display Message")) -> (w646:T75)
        n277 = Enqueue Element(queue=w643, element=w646, error in (no error)=w637) -> (error out=w645:errorcluster)  [unwired: 1 in, 2 out]
      }
      frame "Lig Bipolar - Footswitch Activate Port" {
        n278 = Bundle By Name(cluster=w662, "Footswitch Cluster.PXI-2565 resource name"=w661) -> (w660:T79)
        n279 = Variant To Data(type=TRUE, Variant=w670) -> (data=w654:bool)  [unwired: 1 in, 1 out]
        n280 = call "FT10_PXI-2565 Connect.vi"("error in (no error)"=w659, "Message Handling Cluster in"=w660) -> ("error out"=w655:errorcluster, "Message Handling Cluster out"=w657:T79)  [unwired: 8 in]
        n281 = call "FT10_PXI-2565 Switch Relay.vi"("Activate?"=w654, "error in (no error)"=w655, "Channel 2"="com10" ("channel 2"), "Channel 1"="ch10" ("channel 1"), "Message Handling Cluster in"=w657) -> ("error out"=w651:errorcluster, "Connected?"=w650:bool, "Message Handling Cluster out"=w656:T79)  [unwired: 4 in]
        n282 = local write "Connected?"(w650) -> ()
        n283 = Merge Errors(w651, w659) -> (w658:errorcluster)
        n284 = Bundle By Name(cluster=T75 {"Message"="", "Message Data"=variant} ("Message Cluster"), "Message"="Update Display", "Message Data"="Lig Bipolar - Footswitch Activate Port" ("Display Message")) -> (w667:T75)
        n285 = Enqueue Element(queue=w664, element=w667, error in (no error)=w658) -> (error out=w666:errorcluster)  [unwired: 1 in, 2 out]
      }
      frame "Lig Seal - Footswitch Activate Port" {
        n286 = Bundle By Name(cluster=w683, "Footswitch Cluster.PXI-2565 resource name"=w682) -> (w681:T79)
        n287 = Variant To Data(type=TRUE, Variant=w691) -> (data=w675:bool)  [unwired: 1 in, 1 out]
        n288 = call "FT10_PXI-2565 Connect.vi"("error in (no error)"=w680, "Message Handling Cluster in"=w681) -> ("error out"=w676:errorcluster, "Message Handling Cluster out"=w678:T79)  [unwired: 8 in]
        n289 = call "FT10_PXI-2565 Switch Relay.vi"("Activate?"=w675, "error in (no error)"=w676, "Channel 2"="com11" ("channel 2"), "Channel 1"="ch11" ("channel 1"), "Message Handling Cluster in"=w678) -> ("error out"=w672:errorcluster, "Connected?"=w671:bool, "Message Handling Cluster out"=w677:T79)  [unwired: 4 in]
        n290 = local write "Connected?"(w671) -> ()
        n291 = Merge Errors(w672, w680) -> (w679:errorcluster)
        n292 = Bundle By Name(cluster=T75 {"Message"="", "Message Data"=variant} ("Message Cluster"), "Message"="Update Display", "Message Data"="Lig Seal - Footswitch Activate Port" ("Display Message")) -> (w688:T75)
        n293 = Enqueue Element(queue=w685, element=w688, error in (no error)=w679) -> (error out=w687:errorcluster)  [unwired: 1 in, 2 out]
      }
      frame "Lig Cut - Footswitch Activate Port" {
        n294 = Bundle By Name(cluster=w704, "Footswitch Cluster.PXI-2565 resource name"=w703) -> (w702:T79)
        n295 = Variant To Data(type=TRUE, Variant=w712) -> (data=w696:bool)  [unwired: 1 in, 1 out]
        n296 = call "FT10_PXI-2565 Connect.vi"("error in (no error)"=w701, "Message Handling Cluster in"=w702) -> ("error out"=w697:errorcluster, "Message Handling Cluster out"=w699:T79)  [unwired: 8 in]
        n297 = call "FT10_PXI-2565 Switch Relay.vi"("Activate?"=w696, "error in (no error)"=w697, "Channel 2"="com12" ("channel 2"), "Channel 1"="ch12" ("channel 1"), "Message Handling Cluster in"=w699) -> ("error out"=w693:errorcluster, "Connected?"=w692:bool, "Message Handling Cluster out"=w698:T79)  [unwired: 4 in]
        n298 = local write "Connected?"(w692) -> ()
        n299 = Merge Errors(w693, w701) -> (w700:errorcluster)
        n300 = Bundle By Name(cluster=T75 {"Message"="", "Message Data"=variant} ("Message Cluster"), "Message"="Update Display", "Message Data"="Lig Cut - Footswitch Activate Port" ("Display Message")) -> (w709:T75)
        n301 = Enqueue Element(queue=w706, element=w709, error in (no error)=w700) -> (error out=w708:errorcluster)  [unwired: 1 in, 2 out]
      }
      frame "Lig Coag - Footswitch Activate Port" {
        n302 = Bundle By Name(cluster=w725, "Footswitch Cluster.PXI-2565 resource name"=w724) -> (w723:T79)
        n303 = Variant To Data(type=TRUE, Variant=w733) -> (data=w717:bool)  [unwired: 1 in, 1 out]
        n304 = call "FT10_PXI-2565 Connect.vi"("error in (no error)"=w722, "Message Handling Cluster in"=w723) -> ("error out"=w718:errorcluster, "Message Handling Cluster out"=w720:T79)  [unwired: 8 in]
        n305 = call "FT10_PXI-2565 Switch Relay.vi"("Activate?"=w717, "error in (no error)"=w718, "Channel 2"="com13" ("channel 2"), "Channel 1"="ch13" ("channel 1"), "Message Handling Cluster in"=w720) -> ("error out"=w714:errorcluster, "Connected?"=w713:bool, "Message Handling Cluster out"=w719:T79)  [unwired: 4 in]
        n306 = local write "Connected?"(w713) -> ()
        n307 = Merge Errors(w714, w722) -> (w721:errorcluster)
        n308 = Bundle By Name(cluster=T75 {"Message"="", "Message Data"=variant} ("Message Cluster"), "Message"="Update Display", "Message Data"="Lig Coag - Footswitch Activate Port" ("Display Message")) -> (w730:T75)
        n309 = Enqueue Element(queue=w727, element=w730, error in (no error)=w721) -> (error out=w729:errorcluster)  [unwired: 1 in, 2 out]
      }
      frame "Mono1 Cut Decrease Power" {
        # "Turn power level down on MONO1 Cut Port"
        n310 = call "FT10_Fornax Mono1 Cut Power Down.vi"("Message Handling Cluster in"=w736) -> ("Message Handling Cluster out"=w734:T79)  [unwired: 10 in]
        n311 = Bundle By Name(cluster=T75 {"Message"="", "Message Data"=variant} ("Message Cluster"), "Message"="Update Display", "Message Data"="\"Mono1 Cut Decrease Power\" pressed" ("L10n_Action 1 Pressed")) -> (w741:T75)
        n312 = call "FT10_Fornax Read and Parse.vi"("Message Handling Cluster in"=w734) -> ("Message Handling Cluster out"=w735:T79)  [unwired: 9 in, 1 out]
        n313 = Enqueue Element(queue=w739, element=w741, error in (no error)=w738) -> (error out=w737:errorcluster)  [unwired: 1 in, 2 out]
      }
      frame "Mono2 Cut Decrease Power" {
        # "Turn power level down on MONO2 Cut Port"
        n314 = call "FT10_Fornax Mono2 Cut Power Down.vi"("Message Handling Cluster in"=w746) -> ("Message Handling Cluster out"=w744:T79)  [unwired: 10 in]
        n315 = Bundle By Name(cluster=T75 {"Message"="", "Message Data"=variant} ("Message Cluster"), "Message"="Update Display", "Message Data"="\"Mono2 Cut Decrease Power\" pressed" ("L10n_Action 1 Pressed")) -> (w751:T75)
        n316 = call "FT10_Fornax Read and Parse.vi"("Message Handling Cluster in"=w744) -> ("Message Handling Cluster out"=w745:T79)  [unwired: 9 in, 1 out]
        n317 = Enqueue Element(queue=w749, element=w751, error in (no error)=w748) -> (error out=w747:errorcluster)  [unwired: 1 in, 2 out]
      }
      frame "Mono1 Coag Decrease Power" {
        # "Turn power level down on MONO1 Coag Port"
        n318 = call "FT10_Fornax Mono1 Coag Power Down.vi"("Message Handling Cluster in"=w756) -> ("Message Handling Cluster out"=w755:T79)  [unwired: 10 in]
        n319 = Bundle By Name(cluster=T75 {"Message"="", "Message Data"=variant} ("Message Cluster"), "Message"="Update Display", "Message Data"="\"Mono1 Coag Decrease Power\" pressed" ("L10n_Action 1 Pressed")) -> (w761:T75)
        n320 = call "FT10_Fornax Read and Parse.vi"("Message Handling Cluster in"=w755) -> ("Message Handling Cluster out"=w754:T79)  [unwired: 9 in, 1 out]
        n321 = Enqueue Element(queue=w759, element=w761, error in (no error)=w758) -> (error out=w757:errorcluster)  [unwired: 1 in, 2 out]
      }
      frame "Mono2 Coag Decrease Power" {
        # "Turn power level down on MONO2 Coag Port"
        n322 = call "FT10_Fornax Mono2 Coag Power Down.vi"("Message Handling Cluster in"=w766) -> ("Message Handling Cluster out"=w765:T79)  [unwired: 10 in]
        n323 = Bundle By Name(cluster=T75 {"Message"="", "Message Data"=variant} ("Message Cluster"), "Message"="Update Display", "Message Data"="\"Mono2 Coag Decrease Power\" pressed" ("L10n_Action 1 Pressed")) -> (w771:T75)
        n324 = call "FT10_Fornax Read and Parse.vi"("Message Handling Cluster in"=w765) -> ("Message Handling Cluster out"=w764:T79)  [unwired: 9 in, 1 out]
        n325 = Enqueue Element(queue=w769, element=w771, error in (no error)=w768) -> (error out=w767:errorcluster)  [unwired: 1 in, 2 out]
      }
      frame "Bipolar Decrease Power" {
        # "Turn power level down on Bipolar Port"
        n326 = call "FT10_Fornax Bipolar Power Down.vi"("Message Handling Cluster in"=w776) -> ("Message Handling Cluster out"=w775:T79)  [unwired: 10 in]
        n327 = Bundle By Name(cluster=T75 {"Message"="", "Message Data"=variant} ("Message Cluster"), "Message"="Update Display", "Message Data"="\"Bipolar Decrease Power\" pressed" ("L10n_Action 1 Pressed")) -> (w781:T75)
        n328 = call "FT10_Fornax Read and Parse.vi"("Message Handling Cluster in"=w775) -> ("Message Handling Cluster out"=w774:T79)  [unwired: 9 in, 1 out]
        n329 = Enqueue Element(queue=w779, element=w781, error in (no error)=w778) -> (error out=w777:errorcluster)  [unwired: 1 in, 2 out]
      }
      frame "Mono1 Cut Increase Power" {
        # "Turn power level up on MONO1 Cut Port"
        n330 = call "FT10_Fornax Mono1 Cut Power Up.vi"("Message Handling Cluster in"=w786) -> ("Message Handling Cluster out"=w785:T79)  [unwired: 10 in]
        n331 = Bundle By Name(cluster=T75 {"Message"="", "Message Data"=variant} ("Message Cluster"), "Message"="Update Display", "Message Data"="\"Mono1 Cut Increase Power\" pressed" ("L10n_Action 1 Pressed")) -> (w791:T75)
        n332 = call "FT10_Fornax Read and Parse.vi"("Message Handling Cluster in"=w785) -> ("Message Handling Cluster out"=w784:T79)  [unwired: 9 in, 1 out]
        n333 = Enqueue Element(queue=w789, element=w791, error in (no error)=w788) -> (error out=w787:errorcluster)  [unwired: 1 in, 2 out]
      }
      frame "Mono2 Cut Increase Power" {
        # "Turn power level up on MONO2 Cut Port"
        n334 = call "FT10_Fornax Mono2 Cut Power Up.vi"("Message Handling Cluster in"=w796) -> ("Message Handling Cluster out"=w795:T79)  [unwired: 10 in]
        n335 = Bundle By Name(cluster=T75 {"Message"="", "Message Data"=variant} ("Message Cluster"), "Message"="Update Display", "Message Data"="\"Mono2 Cut Increase Power\" pressed" ("L10n_Action 1 Pressed")) -> (w801:T75)
        n336 = call "FT10_Fornax Read and Parse.vi"("Message Handling Cluster in"=w795) -> ("Message Handling Cluster out"=w794:T79)  [unwired: 9 in, 1 out]
        n337 = Enqueue Element(queue=w799, element=w801, error in (no error)=w798) -> (error out=w797:errorcluster)  [unwired: 1 in, 2 out]
      }
      frame "Mono1 Coag Increase Power" {
        # "Turn power level up on MONO1 Coag Port"
        n338 = call "FT10_Fornax Mono1 Coag Power Up.vi"("Message Handling Cluster in"=w806) -> ("Message Handling Cluster out"=w805:T79)  [unwired: 10 in]
        n339 = Bundle By Name(cluster=T75 {"Message"="", "Message Data"=variant} ("Message Cluster"), "Message"="Update Display", "Message Data"="\"Mono1 Coag Increase Power\" pressed" ("L10n_Action 1 Pressed")) -> (w811:T75)
        n340 = call "FT10_Fornax Read and Parse.vi"("Message Handling Cluster in"=w805) -> ("Message Handling Cluster out"=w804:T79)  [unwired: 9 in, 1 out]
        n341 = Enqueue Element(queue=w809, element=w811, error in (no error)=w808) -> (error out=w807:errorcluster)  [unwired: 1 in, 2 out]
      }
      frame "Mono2 Coag Increase Power" {
        # "Turn power level up on MONO2 Coag Port"
        n342 = call "FT10_Fornax Mono2 Coag Power Up.vi"("Message Handling Cluster in"=w816) -> ("Message Handling Cluster out"=w815:T79)  [unwired: 10 in]
        n343 = Bundle By Name(cluster=T75 {"Message"="", "Message Data"=variant} ("Message Cluster"), "Message"="Update Display", "Message Data"="\"Mono2 Coag Increase Power\" pressed" ("L10n_Action 1 Pressed")) -> (w821:T75)
        n344 = call "FT10_Fornax Read and Parse.vi"("Message Handling Cluster in"=w815) -> ("Message Handling Cluster out"=w814:T79)  [unwired: 9 in, 1 out]
        n345 = Enqueue Element(queue=w819, element=w821, error in (no error)=w818) -> (error out=w817:errorcluster)  [unwired: 1 in, 2 out]
      }
      frame "Bipolar Increase Power" {
        # "Turn power level up on Bipolar Port"
        n346 = call "FT10_Fornax Bipolar Power Up.vi"("Message Handling Cluster in"=w826) -> ("Message Handling Cluster out"=w825:T79)  [unwired: 10 in]
        n347 = Bundle By Name(cluster=T75 {"Message"="", "Message Data"=variant} ("Message Cluster"), "Message"="Update Display", "Message Data"="\"Bipolar Increase Power\" pressed" ("L10n_Action 1 Pressed")) -> (w831:T75)
        n348 = call "FT10_Fornax Read and Parse.vi"("Message Handling Cluster in"=w825) -> ("Message Handling Cluster out"=w824:T79)  [unwired: 9 in, 1 out]
        n349 = Enqueue Element(queue=w829, element=w831, error in (no error)=w828) -> (error out=w827:errorcluster)  [unwired: 1 in, 2 out]
      }
      frame "Mono1 Cut Mode" {
        # "Change mode on MONO1 Cut Port"
        n350 = global read "Abort Auto Test Global.vi" "Abort Auto Test"() -> (w834:bool)
        n351 = Variant To Data(type=Control_Fornax_Mono1_Cut_Enum."Pure" ("Mono1 Cut Enum"), Variant=w840) -> (data=w839:T15)  [unwired: 1 in, 1 out]
        n352 = call "FT10_Fornax Mono1 Cut Mode Command.vi"("Mono1 Cut Enum in"=w839) -> ("Mono1 Cut Enum out"=w835:T15, "JSON Command"=w838:string)  [unwired: 9 in]
        n353 = case shown="False" w834 {
          tunnel: w842 -> [w855 w856]
          tunnel: w838 -> [w851 _]
          tunnel: [w850 w856] -> w837
          frame False {
            n354 = Unbundle By Name(w855) -> ("Fornax Connection"=w853:refnum<k5>)
            n355 = TCP Write(connection ID=w853, data in=w851, 9:100 ("timeout ms (25000)")) -> (connection ID out=w852:refnum<k5>)  [unwired: 1 in, 2 out]
            n356 = Bundle By Name(cluster=w855, "Fornax Connection"=w852) -> (w850:T79)
          }
          frame True {
          }
        }
        n357 = Bundle By Name(cluster=w837, "Log - Port Mode Cluster.Mono1 Cut Enum"=w835) -> (w836:T79)
        n358 = Bundle By Name(cluster=T75 {"Message"="", "Message Data"=variant} ("Message Cluster"), "Message"="Update Display", "Message Data"="\"Mono1 Cut Mode\" pressed" ("L10n_Action 1 Pressed")) -> (w847:T75)
        n359 = Enqueue Element(queue=w845, element=w847, error in (no error)=w844) -> (error out=w843:errorcluster)  [unwired: 1 in, 2 out]
      }
      frame "Mono2 Cut Mode" {
        # "Change mode on MONO2 Cut Port"
        n360 = global read "Abort Auto Test Global.vi" "Abort Auto Test"() -> (w857:bool)
        n361 = Variant To Data(type=Control_Fornax_Mono2_Cut_Enum."Pure" ("Mono2 Cut Enum"), Variant=w862) -> (data=w861:T25)  [unwired: 1 in, 1 out]
        n362 = call "FT10_Fornax Mono2 Cut Mode Command.vi"("Mono2 Cut Enum in"=w861) -> ("Mono2 Cut Enum out"=w858:T25, "JSON Command"=w860:string)  [unwired: 9 in]
        n363 = case shown="False" w857 {
          tunnel: w865 -> [w878 w879]
          tunnel: [w877 w879] -> w864
          tunnel: w860 -> [w873 _]
          frame False {
            n364 = Unbundle By Name(w878) -> ("Fornax Connection"=w875:refnum<k5>)
            n365 = TCP Write(connection ID=w875, data in=w873, 9:100 ("timeout ms (25000)")) -> (connection ID out=w874:refnum<k5>)  [unwired: 1 in, 2 out]
            n366 = Bundle By Name(cluster=w878, "Fornax Connection"=w874) -> (w877:T79)
          }
          frame True {
          }
        }
        n367 = Bundle By Name(cluster=w864, "Log - Port Mode Cluster.Mono2 Cut Enum"=w858) -> (w859:T79)
        n368 = Bundle By Name(cluster=T75 {"Message"="", "Message Data"=variant} ("Message Cluster"), "Message"="Update Display", "Message Data"="\"Mono2 Cut Mode\" pressed" ("L10n_Action 1 Pressed")) -> (w870:T75)
        n369 = Enqueue Element(queue=w868, element=w870, error in (no error)=w867) -> (error out=w866:errorcluster)  [unwired: 1 in, 2 out]
      }
      frame "Mono1 Coag Mode" {
        # "Change mode on MONO1 Coag Port"
        n370 = global read "Abort Auto Test Global.vi" "Abort Auto Test"() -> (w880:bool)
        n371 = Variant To Data(type=Control_Fornax_Mono1_Coag_Enum."Fulgerate" ("Mono1 Coag Enum"), Variant=w885) -> (data=w884:T18)  [unwired: 1 in, 1 out]
        n372 = call "FT10_Fornax Mono1 Coag Mode Command.vi"("Mono1 Coag Enum in"=w884) -> ("Mono1 Coag Enum out"=w881:T18, "JSON Command"=w883:string)  [unwired: 9 in]
        n373 = case shown="False" w880 {
          tunnel: w888 -> [w901 w902]
          tunnel: [w900 w902] -> w887
          tunnel: w883 -> [w896 _]
          frame False {
            n374 = Unbundle By Name(w901) -> ("Fornax Connection"=w898:refnum<k5>)
            n375 = TCP Write(connection ID=w898, data in=w896, 9:100 ("timeout ms (25000)")) -> (connection ID out=w897:refnum<k5>)  [unwired: 1 in, 2 out]
            n376 = Bundle By Name(cluster=w901, "Fornax Connection"=w897) -> (w900:T79)
          }
          frame True {
          }
        }
        n377 = Bundle By Name(cluster=w887, "Log - Port Mode Cluster.Mono1 Coag Enum"=w881) -> (w882:T79)
        n378 = Bundle By Name(cluster=T75 {"Message"="", "Message Data"=variant} ("Message Cluster"), "Message"="Update Display", "Message Data"="\"Mono1 Coag Mode\" pressed" ("L10n_Action 1 Pressed")) -> (w893:T75)
        n379 = Enqueue Element(queue=w891, element=w893, error in (no error)=w890) -> (error out=w889:errorcluster)  [unwired: 1 in, 2 out]
      }
      frame "Mono2 Coag Mode" {
        # "Change mode on MONO2 Coag Port"
        n380 = global read "Abort Auto Test Global.vi" "Abort Auto Test"() -> (w903:bool)
        n381 = Variant To Data(type=Control_Fornax_Mono2_Coag_Enum."Fulgerate" ("Mono2 Coag Enum"), Variant=w908) -> (data=w907:T27)  [unwired: 1 in, 1 out]
        n382 = call "FT10_Fornax Mono2 Coag Mode Command.vi"("Mono2 Coag Enum in"=w907) -> ("Mono2 Coag Enum out"=w904:T27, "JSON Command"=w906:string)  [unwired: 9 in]
        n383 = case shown="False" w903 {
          tunnel: w911 -> [w924 w925]
          tunnel: [w923 w925] -> w910
          tunnel: w906 -> [w919 _]
          frame False {
            n384 = Unbundle By Name(w924) -> ("Fornax Connection"=w921:refnum<k5>)
            n385 = TCP Write(connection ID=w921, data in=w919, 9:100 ("timeout ms (25000)")) -> (connection ID out=w920:refnum<k5>)  [unwired: 1 in, 2 out]
            n386 = Bundle By Name(cluster=w924, "Fornax Connection"=w920) -> (w923:T79)
          }
          frame True {
          }
        }
        n387 = Bundle By Name(cluster=w910, "Log - Port Mode Cluster.Mono2 Coag Enum"=w904) -> (w905:T79)
        n388 = Bundle By Name(cluster=T75 {"Message"="", "Message Data"=variant} ("Message Cluster"), "Message"="Update Display", "Message Data"="\"Mono2 Coag Mode\" pressed" ("L10n_Action 1 Pressed")) -> (w916:T75)
        n389 = Enqueue Element(queue=w914, element=w916, error in (no error)=w913) -> (error out=w912:errorcluster)  [unwired: 1 in, 2 out]
      }
      frame "Bipolar Mode" {
        # "Change mode on Bipolar Port"
        n390 = global read "Abort Auto Test Global.vi" "Abort Auto Test"() -> (w926:bool)
        n391 = Variant To Data(type=Control_Fornax_Bipolar_Enum."Standard" ("Bipolar Enum"), Variant=w931) -> (data=w930:T13)  [unwired: 1 in, 1 out]
        n392 = call "FT10_Fornax Bipolar Mode Command.vi"("Bipolar Enum in"=w930) -> ("Bipolar Enum out"=w927:T13, "JSON Command"=w929:string)  [unwired: 9 in]
        n393 = case shown="False" w926 {
          tunnel: w934 -> [w947 w948]
          tunnel: [w946 w948] -> w933
          tunnel: w929 -> [w942 _]
          frame False {
            n394 = Unbundle By Name(w947) -> ("Fornax Connection"=w944:refnum<k5>)
            n395 = TCP Write(connection ID=w944, data in=w942, 9:100 ("timeout ms (25000)")) -> (connection ID out=w943:refnum<k5>)  [unwired: 1 in, 2 out]
            n396 = Bundle By Name(cluster=w947, "Fornax Connection"=w943) -> (w946:T79)
          }
          frame True {
          }
        }
        n397 = Bundle By Name(cluster=w933, "Log - Port Mode Cluster.Bipolar Enum"=w927) -> (w928:T79)
        n398 = Bundle By Name(cluster=T75 {"Message"="", "Message Data"=variant} ("Message Cluster"), "Message"="Update Display", "Message Data"="\"Bipolar Mode\" pressed" ("L10n_Action 1 Pressed")) -> (w939:T75)
        n399 = Enqueue Element(queue=w937, element=w939, error in (no error)=w936) -> (error out=w935:errorcluster)  [unwired: 1 in, 2 out]
      }
      frame "Wait" {
        # "Wait for specified time (ms)"
        n400 = global read "Abort Auto Test Global.vi" "Abort Auto Test"() -> (w949:bool)
        n401 = case shown="False" w949 {
          tunnel: w951 -> [w961 _]
          frame False {
            n402 = Variant To Data(type=0 ("Wait Time (ms)"), Variant=w961) -> (data=w959:i32)  [unwired: 1 in, 1 out]
            n403 = Wait (ms)(milliseconds to wait=w959) -> ()  [unwired: 1 out]
          }
          frame True {
          }
        }
        n404 = Bundle By Name(cluster=T75 {"Message"="", "Message Data"=variant} ("Message Cluster"), "Message"="Update Display", "Message Data"="\"Wait\" pressed" ("L10n_Action 1 Pressed")) -> (w956:T75)
        n405 = Enqueue Element(queue=w954, element=w956, error in (no error)=w953) -> (error out=w952:errorcluster)  [unwired: 1 in, 2 out]
      }
      frame "Log?" {
        # "Update Log Flag"
        n406 = Variant To Data(type=T87 FALSE ("Log Flag"), Variant=w966) -> (data=w963:T87)  [unwired: 1 in, 1 out]
        n407 = Bundle By Name(cluster=w965, "Log Flag"=w963) -> (w964:T79)
      }
      frame "Update Display" {
        # "Update Display - Convert the Message Data to a string to display in the Display Message indicator."
        n408 = Variant To Data(error in=w973, type="", Variant=w972) -> (data=→"Display Message":string, error out=w970:errorcluster)
      }
      frame "Exit" {
        # "Release the message queue reference."
        # "Exit - Exit the application. Since this message was sent as a priority message (i.e., it was placed at the front of the queue), any cleanup code should run here, since the loop is about to stop. Any other messages in the queue will not be handled."
        n409 = Unbundle By Name(w983) -> ("UNITHERM Connection"=w985:refnum<visa-resource-name>, "FPGA VI Reference Out"=w977:T81)
        n410 = Release Queue(queue=w988, error in (no error)=w981) -> (error out=w987:errorcluster)  [unwired: 1 in, 2 out]
        n411 = call "FT10_Unitherm Clear Load.vi"("error in (no error)"=w981, "VISA Refnum in"=w985) -> ("error out"=w975:errorcluster, "VISA Refnum out"=w984:refnum<visa-resource-name>)  [unwired: 7 in, 1 out]
        n412 = call "FT10_FPGA_7854R Set Relay Config.vi"("Update Config Enum"=T99."Off", "Refnum in"=w977) -> ("Refnum out"=w976:T81)  [unwired: 9 in]
        n413 = Merge Errors(w975, w987) -> (w979:errorcluster)
        n414 = Bundle By Name(cluster=w983, "UNITHERM Connection"=w984, "FPGA VI Reference Out"=w976) -> (w982:T79)
        n415 = flat-sequence {
          tunnel: w979 -> [w989]
          tunnel: [w989] -> w978
          frame #0 {
            n416 = call "FT10_Stop Notifier.vi"("Selector"=Config_Stop_Notifier_Enum."Notify") -> ()  [unwired: 9 in, 2 out]
          }
        }
        n417 = local write "Display Message"("\"Stop\" button pressed" ("L10n_Stop Pressed")) -> ()
      }
      frame Default {
        # "The Default case only runs if there is a message that isn't defined in any of the other cases. Generate an error if this occurs."
        n418 = xnode "Error Ring"("parameter 0"=w994) -> ("error out"=w992:errorcluster)
        n419 = call <vilib>:"Simple Error Handler.vi"("error in (no error)"=w992) -> ()  [unwired: 4 in, 5 out]
      }
    }
  }
  n420 = while {
    tunnel: w11 -> [w1012]
    tunnel: w8 -> [w1011]
    tunnel: [w1008] -> w6
    tunnel: [w1007] -> w7
    shift-right: [w1005] -> _
    shift-left: T59 {"tdms file out"=refnum, "t0"="", "Generator Serial Number in"="T1234567DX"} -> [w1004]
    tunnel: w2 -> [w1002]
    stop <- w1003 stop-if-true
    # "Logging Loop"
    n421 = Get Queue Status(queue=w1012, error in (no error)=w1011) -> (queue out=w1010:refnum<queue>, error out=w1009:errorcluster, # elements in queue=w1013:i32)  [unwired: 1 in, 5 out]
    n422 = Not Equal To 0?(x=w1013) -> (x != 0?=w1006:bool)
    "Logging?" <- w1006
    n423 = case shown="True" w1006 {
      tunnel: w1010 -> [w1016 w1020]
      tunnel: w1009 -> [w1015 w1018]
      tunnel: [w1016 w1031] -> w1008
      tunnel: [w1015 w1030] -> w1007
      tunnel: [w1014 w1029] -> w1005
      tunnel: w1004 -> [w1014 w1022]
      tunnel: w1002 -> [_ w1017]
      frame False {
        # "Do Nothing"
      }
      frame True {
        # "Log Values"
        n424 = First Call?() -> (First Call?: T/F=w1024:bool)
        n425 = case shown="True" w1024 {
          tunnel: [w1034 w1037] -> w1023
          tunnel: w1022 -> [w1034 w1038]
          tunnel: [w1033 w1036] -> w1021
          tunnel: w1020 -> [w1033 w1036]
          tunnel: [w1032 w1041] -> w1019
          tunnel: w1018 -> [w1032 w1041]
          tunnel: w1017 -> [_ w1035]
          frame False {
          }
          frame True {
            n426 = call "FT10_Log Create TDMS File.vi"("Generator Serial Number in"=w1035) -> ("t0"=w1039:T61, "tdms file out"=w1040:T60)  [unwired: 9 in]
            n427 = Bundle By Name(cluster=w1038, "tdms file out"=w1040, "t0"=w1039, "Generator Serial Number in"=w1035) -> (w1037:T59)
          }
        }
        n428 = Dequeue Element(queue=w1021, error in (no error)=w1019) -> (queue out=w1031:refnum<queue>, element=w1028:T64, error out=w1030:errorcluster)  [unwired: 1 in, 1 out]
        n429 = call "FT10_Log LVM Values.vi"("Log Cluster in"=w1028, "Log Loop Cluster in"=w1023) -> ("Filename Cluster out"=w1025:T101, "Log Cluster out"=w1026:T64, "Log Loop Cluster out"=w1027:T59)  [unwired: 6 in, 1 out]
        n430 = call "FT10_Log TDMS Values.vi"("Filename Cluster in"=w1025, "Log Cluster in"=w1026, "Log Loop Cluster in"=w1027) -> ("Log Loop Cluster out"=w1029:T59)  [unwired: 7 in, 1 out]
      }
    }
    n431 = call "FT10_Read Stop Notifier.vi"() -> ("Stop Notifier"=w1003:bool)  [unwired: 10 in, 1 out]
  }
  n432 = while {
    tunnel: w19 -> [w1049]
    tunnel: [w1048] -> w27
    shift-right: [w1045] -> _
    shift-left: _ -> [w1047]
    tunnel: [w1044] -> w1
    shift-right: [w1043] -> _
    shift-left: _ -> [w1042]
    stop <- w1046 stop-if-true
    # "Event Handling Loop"
    n433 = event shown="[52] \"Run Semi-Auto 2 Commands\": Value Change" {
      selector: _ -> [_ _ _ _ _ _ _ _ _ _ _ _ _ _ _ _ _ _ _ _ _ _ _ _ _ _ _ _ _ _ _ _ _ _ _ _ _ _ _ _ _ _ _ _ _ _ _ _ _ _ _ _ _ _ _]
      dyn-events: _ -> [_ _ _ _ _ _ _ _ _ _ _ _ _ _ _ _ _ _ _ _ _ _ _ _ _ _ _ _ _ _ _ _ _ _ _ _ _ _ _ _ _ _ _ _ _ _ _ _ _ _ _ _ _ _ _]
      timeout: _ -> [_ _ _ _ _ _ _ _ _ _ _ _ _ _ _ _ _ _ _ _ _ _ _ _ _ _ _ _ _ _ _ _ _ _ _ _ _ _ _ _ _ _ _ _ _ _ _ _ _ _ _ _ _ _ _]
      tunnel: [_ _ _ _ _ _ _ _ _ _ _ _ _ _ _ _ _ _ _ _ _ _ _ _ _ _ _ _ _ _ _ _ _ _ _ _ _ _ _ _ _ _ _ _ _ _ _ _ _ _ _ FALSE _ w1574 TRUE] -> w1046
      tunnel: w1049 -> [w1058 w1069 w1079 w1091 w1099 w1116 w1136 w1144 w1148 w1170 w1181 w1192 w1203 w1214 w1225 w1236 w1247 w1258 w1269 w1279 w1287 w1295 w1303 w1311 w1320 w1331 w1342 w1353 w1364 w1375 w1385 w1393 w1401 w1409 w1417 w1425 w1433 w1441 w1449 w1457 w1465 w1473 w1481 w1489 w1497 w1505 w1513 w1521 w1529 _ w1542 _ w1562 w1576 w1581]
      tunnel: [w1057 w1068 w1078 w1090 w1100 w1115 w1135 w1143 w1150 w1171 w1182 w1193 w1204 w1215 w1226 w1237 w1248 w1259 w1270 w1280 w1288 w1296 w1304 w1312 w1321 w1332 w1343 w1354 w1365 w1376 w1386 w1394 w1402 w1410 w1418 w1426 w1434 w1442 w1450 w1458 w1466 w1474 w1482 w1490 w1498 w1506 w1514 w1522 w1530 _ _ _ _ w1578 w1584] -> w1048
      tunnel: [w1051 w1062 w1073 w1082 w1095 w1112 w1130 w1138 w1146 w1167 w1178 w1189 w1200 w1211 w1222 w1235 w1246 w1257 w1268 w1278 w1286 w1294 w1302 w1310 w1319 w1330 w1341 w1352 w1363 w1374 w1384 w1392 w1400 w1408 w1415 w1423 w1431 w1439 w1447 w1455 w1463 w1471 w1479 w1487 w1495 w1503 w1511 w1519 w1527 w1536 w1541 w1555 w1561 w1575 w1580] -> w1045
      tunnel: w1047 -> [w1051 w1062 w1073 w1082 w1095 w1112 w1130 w1138 w1146 w1167 w1178 w1189 w1200 w1211 w1222 w1235 w1246 w1257 w1268 w1278 w1286 w1294 w1302 w1310 w1319 w1330 w1341 w1352 w1363 w1374 w1384 w1392 w1400 w1408 w1415 w1423 w1431 w1439 w1447 w1455 w1463 w1471 w1479 w1487 w1495 w1503 w1511 w1519 w1527 _ w1541 w1555 w1561 w1575 w1580]
      tunnel: [_ _ _ _ _ _ _ _ _ _ _ _ _ _ _ _ _ _ _ _ _ _ _ _ _ _ _ _ _ _ _ _ _ _ _ _ _ _ _ _ _ _ _ _ _ _ _ _ _ _ _ _ _ w1574 _] -> w1044
      tunnel: [w1050 w1061 w1072 w1080 w1094 w1111 w1129 w1137 w1145 w1166 w1177 w1188 w1199 w1210 w1221 w1232 w1243 w1254 w1265 w1277 w1285 w1293 w1301 w1309 w1316 w1327 w1338 w1349 w1360 w1371 w1383 w1391 w1399 w1407 w1414 w1422 w1430 w1438 w1446 w1454 w1462 w1470 w1478 w1486 w1494 w1502 w1510 w1518 w1526 w1534 w1540 w1553 w1560 w1573 w1579] -> w1043
      tunnel: w1042 -> [w1050 w1061 w1072 w1080 w1094 w1111 w1129 w1137 w1145 w1166 w1177 w1188 w1199 w1210 w1221 w1232 w1243 w1254 w1265 w1277 w1285 w1293 w1301 w1309 w1316 w1327 w1338 w1349 w1360 w1371 w1383 w1391 w1399 w1407 w1414 w1422 w1430 w1438 w1446 w1454 w1462 w1470 w1478 w1486 w1494 w1502 w1510 w1518 w1526 w1534 w1540 _ w1560 w1573 w1579]
      event Value Change {
        # "Enqueue an \"Action 1\" message."
        n434 = event-data() -> ()  [unwired: 1 in, 1 out]
        n435 = case shown="True" "Fornax Connect/Disconnect" {
          tunnel: ["Connect" ("Boolean Text.Text") "Disconnect" ("Boolean Text.Text")] -> w1052
          frame False {
          }
          frame True {
          }
        }
        n436 = property on="Fornax Connect/Disconnect" class="Bool (strict)"("BoolText.Text"=w1052) -> ()  [unwired: 2 in, 2 out]
        n437 = Bundle By Name(cluster=T75 {"Message"="Fornax Connect/Disconnect", "Message Data"=variant} ("element"), "Message"="Fornax Connect/Disconnect", "Message Data"="Fornax Connect/Disconnect") -> (w1054:T75)
        n438 = Enqueue Element(queue=w1058, element=w1054) -> (error out=w1057:errorcluster)  [unwired: 2 in, 2 out]
      }
      event Value Change {
        # "Enqueue an \"Action 1\" message."
        n439 = event-data() -> ()  [unwired: 1 in, 1 out]
        n440 = case shown="True" "M4X Connect/Disconnect" {
          tunnel: ["Connect" ("Boolean Text.Text") "Disconnect" ("Boolean Text.Text")] -> w1063
          frame False {
          }
          frame True {
          }
        }
        n441 = property on="M4X Connect/Disconnect" class="Bool (strict)"("BoolText.Text"=w1063) -> ()  [unwired: 2 in, 2 out]
        n442 = Bundle By Name(cluster=T75 {"Message"="Fornax Connect/Disconnect", "Message Data"=variant} ("element"), "Message"="M4X Connect/Disconnect", "Message Data"="M4X Connect/Disconnect") -> (w1065:T75)
        n443 = Enqueue Element(queue=w1069, element=w1065) -> (error out=w1068:errorcluster)  [unwired: 2 in, 2 out]
      }
      event Value Change {
        # "Enqueue an \"Action 1\" message."
        n444 = event-data() -> ()  [unwired: 1 in, 1 out]
        n445 = Bundle By Name(cluster=T75 {"Message"="Fornax Connect/Disconnect", "Message Data"=variant} ("element"), "Message"="Log?", "Message Data"="Log?") -> (w1075:T75)
        n446 = Enqueue Element(queue=w1079, element=w1075) -> (error out=w1078:errorcluster)  [unwired: 2 in, 2 out]
      }
      event Value Change {
        # "Enqueue an \"Action 1\" message."
        n447 = event-data() -> ()  [unwired: 1 in, 1 out]
        n448 = Bundle By Name(cluster=T96 {"Unitherm Connect/Disconnect"=FALSE, "Unitherm Refnum in"=""}, "Unitherm Connect/Disconnect"="Unitherm Connect/Disconnect", "Unitherm Refnum in"="Unitherm Refnum in") -> (w1086:T96)
        n449 = case shown="True" "Unitherm Connect/Disconnect" {
          tunnel: ["Connect" ("Boolean Text.Text") "Disconnect" ("Boolean Text.Text")] -> w1083
          frame False {
          }
          frame True {
          }
        }
        n450 = property on="Unitherm Connect/Disconnect" class="Bool (strict)"("BoolText.Text"=w1083) -> ()  [unwired: 2 in, 2 out]
        n451 = Bundle By Name(cluster=T75 {"Message"="Fornax Connect/Disconnect", "Message Data"=variant} ("element"), "Message"="Unitherm Connect/Disconnect", "Message Data"=w1086) -> (w1087:T75)
        n452 = Enqueue Element(queue=w1091, element=w1087) -> (error out=w1090:errorcluster)  [unwired: 2 in, 2 out]
      }
      event Value Change {
        n453 = event-data() -> ()  [unwired: 1 in, 1 out]
        n454 = Bundle By Name(cluster=T97 {"PXI-7854R Resource"="PXI1Slot6", "75kHz"=TRUE, "uSec Off"=6, "uSec On"=7, "7854 Connect/Disconnect"=FALSE}, "7854 Connect/Disconnect"="7854 Connect/Disconnect", "75kHz"="75kHz", "uSec Off"="uSec Off", "uSec On"="uSec On", "PXI-7854R Resource"="resource name") -> (w1101:T97)
        n455 = case shown="True" "7854 Connect/Disconnect" {
          tunnel: ["Connect" ("Boolean Text.Text") "Disconnect" ("Boolean Text.Text")] -> w1097
          frame False {
          }
          frame True {
          }
        }
        n456 = property on="7854 Connect/Disconnect" class="Bool (strict)"("BoolText.Text"=w1097) -> ()  [unwired: 2 in, 2 out]
        n457 = Bundle By Name(cluster=T75 {"Message"="Fornax Connect/Disconnect", "Message Data"=variant} ("element"), "Message"="7854 Connect/Disconnect", "Message Data"=w1101) -> (w1107:T75)
        n458 = Enqueue Element(queue=w1099, element=w1107) -> (error out=w1100:errorcluster)  [unwired: 2 in, 2 out]
      }
      event Value Change {
        # "Enqueue an \"Action 1\" message."
        n459 = event-data() -> ()  [unwired: 1 in, 1 out]
        n460 = disable-structure shown="Disabled" {
          frame Disabled {
            n461 = call "FT10_Unitherm Ask Dialog - Set Load.vi"() -> ()  [unwired: 11 in, 1 out]
          }
          frame Enabled {
          }
        }
        n462 = case shown="True" "Set Load" {
          tunnel: w1116 -> [w1122 w1128]
          tunnel: [w1118 w1124] -> w1115
          tunnel: "Load (Ohms)" -> [w1117 _]
          frame True {
            n463 = Bundle By Name(cluster=T75 {"Message"="Fornax Connect/Disconnect", "Message Data"=variant} ("element"), "Message"="Set Load", "Message Data"=w1117) -> (w1119:T75)
            n464 = Enqueue Element(queue=w1122, element=w1119) -> (error out=w1118:errorcluster)  [unwired: 2 in, 2 out]
          }
          frame False {
            n465 = Bundle By Name(cluster=T75 {"Message"="Fornax Connect/Disconnect", "Message Data"=variant} ("element"), "Message"="Update Display", "Message Data"="Unitherm Set Load Canceled" ("Message")) -> (w1125:T75)
            n466 = Enqueue Element(queue=w1128, element=w1125) -> (error out=w1124:errorcluster)  [unwired: 2 in, 2 out]
          }
        }
      }
      event Value Change {
        # "Enqueue an \"Action 1\" message."
        n467 = event-data() -> ()  [unwired: 1 in, 1 out]
        n468 = Bundle By Name(cluster=T75 {"Message"="Fornax Connect/Disconnect", "Message Data"=variant} ("element"), "Message"="Clear Load", "Message Data"="Clear Load") -> (w1132:T75)
        n469 = Enqueue Element(queue=w1136, element=w1132) -> (error out=w1135:errorcluster)  [unwired: 2 in, 2 out]
      }
      event Value Change {
        # "Enqueue an \"Action 1\" message."
        n470 = event-data() -> ()  [unwired: 1 in, 1 out]
        n471 = Bundle By Name(cluster=T75 {"Message"="Fornax Connect/Disconnect", "Message Data"=variant} ("element"), "Message"="Read Current", "Message Data"="Read Current") -> (w1140:T75)
        n472 = Enqueue Element(queue=w1144, element=w1140) -> (error out=w1143:errorcluster)  [unwired: 2 in, 2 out]
      }
      event Value Change {
        n473 = event-data() -> ()  [unwired: 1 in, 1 out]
        n474 = disable-structure shown="Disabled" {
          frame Disabled {
            n475 = call "FT10_FPGA_7854R Ask Dialog - Set Config.vi"() -> ()  [unwired: 11 in, 1 out]
          }
          frame Enabled {
          }
        }
        n476 = case shown="True" "7854 Set Config" {
          selector: "7854 Set Config" -> [_ w1158]
          tunnel: [w1151 w1160] -> w1150
          tunnel: "7854 Config Enum" -> [_ w1159]
          tunnel: w1148 -> [w1152 w1157]
          frame False {
            n477 = Bundle By Name(cluster=T75 {"Message"="Fornax Connect/Disconnect", "Message Data"=variant} ("element"), "Message"="Update Display", "Message Data"="PXI-7854R Set Configuration Canceled" ("Message")) -> (w1156:T75)
            n478 = Enqueue Element(queue=w1152, element=w1156) -> (error out=w1151:errorcluster)  [unwired: 2 in, 2 out]
          }
          frame True {
            n479 = Bundle By Name(cluster=T98 {"7854 Config Enum"=enum."Mono 1", "7854 Set Config"=FALSE}, "7854 Config Enum"=w1159, "7854 Set Config"=w1158) -> (w1161:T98)
            n480 = Bundle By Name(cluster=T75 {"Message"="Fornax Connect/Disconnect", "Message Data"=variant} ("element"), "Message"="7854 Set Config", "Message Data"=w1161) -> (w1164:T75)
            n481 = Enqueue Element(queue=w1157, element=w1164) -> (error out=w1160:errorcluster)  [unwired: 2 in, 2 out]
          }
        }
      }
      event Value Change {
        # "Turn power ON or OFF on MONO1 Cut Port"
        n482 = event-data() -> ()  [unwired: 1 in, 1 out]
        n483 = case shown="True" "Mono1 Cut Activate" {
          tunnel: ["Deactivate" ("Message") "Activate" ("Message")] -> w1168
          frame True {
          }
          frame False {
          }
        }
        n484 = property on="Mono1 Cut Activate" class="Bool (strict)"("BoolText.Text"=w1168) -> ()  [unwired: 2 in, 2 out]
        n485 = Bundle By Name(cluster=T75 {"Message"="", "Message Data"=variant} ("element"), "Message Data"="Mono1 Cut Activate", "Message"="Mono1 Cut Activate Port") -> (w1173:T75)
        n486 = Enqueue Element(queue=w1170, element=w1173) -> (error out=w1171:errorcluster)  [unwired: 2 in, 2 out]
      }
      event Value Change {
        # "Turn power ON or OFF on MONO2 Cut Port"
        n487 = event-data() -> ()  [unwired: 1 in, 1 out]
        n488 = case shown="True" "Mono2 Cut Activate" {
          tunnel: ["Deactivate" ("Message") "Activate" ("Message")] -> w1179
          frame True {
          }
          frame False {
          }
        }
        n489 = property on="Mono2 Cut Activate" class="Bool (strict)"("BoolText.Text"=w1179) -> ()  [unwired: 2 in, 2 out]
        n490 = Bundle By Name(cluster=T75 {"Message"="", "Message Data"=variant} ("element"), "Message Data"="Mono2 Cut Activate", "Message"="Mono2 Cut Activate Port") -> (w1184:T75)
        n491 = Enqueue Element(queue=w1181, element=w1184) -> (error out=w1182:errorcluster)  [unwired: 2 in, 2 out]
      }
      event Value Change {
        # "Turn power ON or OFF on MONO1 Coag Port"
        n492 = event-data() -> ()  [unwired: 1 in, 1 out]
        n493 = case shown="True" "Mono1 Coag Activate" {
          tunnel: ["Deactivate" ("Message") "Activate" ("Message")] -> w1190
          frame True {
          }
          frame False {
          }
        }
        n494 = property on="Mono1 Coag Activate" class="Bool (strict)"("BoolText.Text"=w1190) -> ()  [unwired: 2 in, 2 out]
        n495 = Bundle By Name(cluster=T75 {"Message"="", "Message Data"=variant} ("element"), "Message Data"="Mono1 Coag Activate", "Message"="Mono1 Coag Activate Port") -> (w1195:T75)
        n496 = Enqueue Element(queue=w1192, element=w1195) -> (error out=w1193:errorcluster)  [unwired: 2 in, 2 out]
      }
      event Value Change {
        # "Turn power ON or OFF on MONO2 Coag Port"
        n497 = event-data() -> ()  [unwired: 1 in, 1 out]
        n498 = case shown="True" "Mono2 Coag Activate" {
          tunnel: ["Deactivate" ("Message") "Activate" ("Message")] -> w1201
          frame True {
          }
          frame False {
          }
        }
        n499 = property on="Mono2 Coag Activate" class="Bool (strict)"("BoolText.Text"=w1201) -> ()  [unwired: 2 in, 2 out]
        n500 = Bundle By Name(cluster=T75 {"Message"="", "Message Data"=variant} ("element"), "Message Data"="Mono2 Coag Activate", "Message"="Mono2 Coag Activate Port") -> (w1206:T75)
        n501 = Enqueue Element(queue=w1203, element=w1206) -> (error out=w1204:errorcluster)  [unwired: 2 in, 2 out]
      }
      event Value Change {
        # "Turn power ON or OFF on Ligasure Port"
        n502 = event-data() -> ()  [unwired: 1 in, 1 out]
        n503 = case shown="True" "Ligasure Activate" {
          tunnel: ["Deactivate" ("Message") "Activate" ("Message")] -> w1213
          frame True {
          }
          frame False {
          }
        }
        n504 = property on="Ligasure Activate" class="Bool (strict)"("BoolText.Text"=w1213) -> ()  [unwired: 2 in, 2 out]
        n505 = Bundle By Name(cluster=T75 {"Message"="", "Message Data"=variant} ("element"), "Message Data"="Ligasure Activate", "Message"="Ligasure Activate Port") -> (w1217:T75)
        n506 = Enqueue Element(queue=w1214, element=w1217) -> (error out=w1215:errorcluster)  [unwired: 2 in, 2 out]
      }
      event Value Change {
        # "Turn power ON or OFF on Bipolar Port"
        n507 = event-data() -> ()  [unwired: 1 in, 1 out]
        n508 = case shown="True" "Bipolar Activate" {
          tunnel: ["Deactivate" ("Message") "Activate" ("Message")] -> w1224
          frame True {
          }
          frame False {
          }
        }
        n509 = property on="Bipolar Activate" class="Bool (strict)"("BoolText.Text"=w1224) -> ()  [unwired: 2 in, 2 out]
        n510 = Bundle By Name(cluster=T75 {"Message"="", "Message Data"=variant} ("element"), "Message Data"="Bipolar Activate", "Message"="Bipolar Activate Port") -> (w1228:T75)
        n511 = Enqueue Element(queue=w1225, element=w1228) -> (error out=w1226:errorcluster)  [unwired: 2 in, 2 out]
      }
      event "Mono1 Cut - Handswitch": Value Change {
        # "Turn power ON or OFF on MONO2 Coag Port"
        n512 = event-data() -> ()  [unwired: 1 in, 1 out]
        n513 = case shown="True" "Mono1 Cut - Handswitch" {
          tunnel: ["Deactivate Cut" ("Message") "Activate Cut" ("Message")] -> w1233
          frame True {
          }
          frame False {
          }
        }
        n514 = property on="Mono1 Cut - Handswitch" class="Bool (strict)"("BoolText.Text"=w1233) -> ()  [unwired: 2 in, 2 out]
        n515 = Bundle By Name(cluster=T75 {"Message"="", "Message Data"=variant} ("element"), "Message Data"="Mono1 Cut - Handswitch", "Message"="Mono1 Cut - Handswitch Activate Port") -> (w1239:T75)
        n516 = Enqueue Element(queue=w1236, element=w1239) -> (error out=w1237:errorcluster)  [unwired: 2 in, 2 out]
      }
      event "Mono1 Coag - Handswitch": Value Change {
        # "Turn power ON or OFF on MONO2 Coag Port"
        n517 = event-data() -> ()  [unwired: 1 in, 1 out]
        n518 = case shown="False" "Mono1 Coag - Handswitch" {
          tunnel: ["Deactivate Coag" ("Message") "Activate Coag" ("Message")] -> w1244
          frame True {
          }
          frame False {
          }
        }
        n519 = property on="Mono1 Coag - Handswitch" class="Bool (strict)"("BoolText.Text"=w1244) -> ()  [unwired: 2 in, 2 out]
        n520 = Bundle By Name(cluster=T75 {"Message"="", "Message Data"=variant} ("element"), "Message Data"="Mono1 Coag - Handswitch", "Message"="Mono1 Coag - Handswitch Activate Port") -> (w1250:T75)
        n521 = Enqueue Element(queue=w1247, element=w1250) -> (error out=w1248:errorcluster)  [unwired: 2 in, 2 out]
      }
      event "Mono2 Cut - Handswitch": Value Change {
        # "Turn power ON or OFF on MONO2 Coag Port"
        n522 = event-data() -> ()  [unwired: 1 in, 1 out]
        n523 = case shown="False" "Mono2 Cut - Handswitch" {
          tunnel: ["Deactivate Cut" ("Message") "Activate Cut" ("Message")] -> w1255
          frame True {
          }
          frame False {
          }
        }
        n524 = property on="Mono2 Cut - Handswitch" class="Bool (strict)"("BoolText.Text"=w1255) -> ()  [unwired: 2 in, 2 out]
        n525 = Bundle By Name(cluster=T75 {"Message"="", "Message Data"=variant} ("element"), "Message Data"="Mono2 Cut - Handswitch", "Message"="Mono2 Cut - Handswitch Activate Port") -> (w1261:T75)
        n526 = Enqueue Element(queue=w1258, element=w1261) -> (error out=w1259:errorcluster)  [unwired: 2 in, 2 out]
      }
      event "Mono2 Coag - Handswitch": Value Change {
        # "Turn power ON or OFF on MONO2 Coag Port"
        n527 = event-data() -> ()  [unwired: 1 in, 1 out]
        n528 = case shown="False" "Mono2 Coag - Handswitch" {
          tunnel: ["Deactivate Coag" ("Message") "Activate Coag" ("Message")] -> w1266
          frame True {
          }
          frame False {
          }
        }
        n529 = property on="Mono2 Coag - Handswitch" class="Bool (strict)"("BoolText.Text"=w1266) -> ()  [unwired: 2 in, 2 out]
        n530 = Bundle By Name(cluster=T75 {"Message"="", "Message Data"=variant} ("element"), "Message Data"="Mono2 Coag - Handswitch", "Message"="Mono2 Coag - Handswitch Activate Port") -> (w1272:T75)
        n531 = Enqueue Element(queue=w1269, element=w1272) -> (error out=w1270:errorcluster)  [unwired: 2 in, 2 out]
      }
      event "Mono2 Triverse Tab": Value Change {
        # "Turn power ON or OFF on MONO2 Coag Port"
        n532 = event-data() -> ()  [unwired: 1 in, 1 out]
        n533 = Bundle By Name(cluster=T75 {"Message"="", "Message Data"=variant} ("element"), "Message Data"="Mono2 Triverse Tab", "Message"="Mono2 Triverse Tab") -> (w1282:T75)
        n534 = Enqueue Element(queue=w1279, element=w1282) -> (error out=w1280:errorcluster)  [unwired: 2 in, 2 out]
      }
      event "Triverse Slide": Value Change {
        # "Turn power ON or OFF on MONO2 Coag Port"
        n535 = event-data() -> ()  [unwired: 1 in, 1 out]
        n536 = Bundle By Name(cluster=T75 {"Message"="", "Message Data"=variant} ("element"), "Message Data"="Triverse Slide", "Message"="Triverse Slide") -> (w1290:T75)
        n537 = Enqueue Element(queue=w1287, element=w1290) -> (error out=w1288:errorcluster)  [unwired: 2 in, 2 out]
      }
      event "Mono2 Triverse - Handswitch Seal": Value Change {
        # "Turn power ON or OFF on MONO2 Coag Port"
        n538 = event-data() -> ()  [unwired: 1 in, 1 out]
        n539 = Bundle By Name(cluster=T75 {"Message"="", "Message Data"=variant} ("element"), "Message Data"="Mono2 Triverse - Handswitch Seal", "Message"="Mono2 Triverse - Handswitch Seal") -> (w1298:T75)
        n540 = Enqueue Element(queue=w1295, element=w1298) -> (error out=w1296:errorcluster)  [unwired: 2 in, 2 out]
      }
      event "Mono2 Triverse - Handswitch Cut": Value Change {
        # "Turn power ON or OFF on MONO2 Coag Port"
        n541 = event-data() -> ()  [unwired: 1 in, 1 out]
        n542 = Bundle By Name(cluster=T75 {"Message"="", "Message Data"=variant} ("element"), "Message Data"="Mono2 Triverse - Handswitch Cut", "Message"="Mono2 Triverse - Handswitch Cut") -> (w1306:T75)
        n543 = Enqueue Element(queue=w1303, element=w1306) -> (error out=w1304:errorcluster)  [unwired: 2 in, 2 out]
      }
      event "Mono2 Triverse - Handswitch Coag": Value Change {
        # "Turn power ON or OFF on MONO2 Coag Port"
        n544 = event-data() -> ()  [unwired: 1 in, 1 out]
        n545 = Bundle By Name(cluster=T75 {"Message"="", "Message Data"=variant} ("element"), "Message Data"="Mono2 Triverse - Handswitch Coag", "Message"="Mono2 Triverse - Handswitch Coag") -> (w1314:T75)
        n546 = Enqueue Element(queue=w1311, element=w1314) -> (error out=w1312:errorcluster)  [unwired: 2 in, 2 out]
      }
      event "Mono1 Cut - Footswitch": Value Change {
        # "Turn power ON or OFF on MONO2 Coag Port"
        n547 = event-data() -> ()  [unwired: 1 in, 1 out]
        n548 = case shown="False" "Mono1 Cut - Footswitch" {
          tunnel: ["Deactivate Cut" ("Message") "Activate Cut" ("Message")] -> w1317
          frame True {
          }
          frame False {
          }
        }
        n549 = property on="Mono1 Cut - Footswitch" class="Bool (strict)"("BoolText.Text"=w1317) -> ()  [unwired: 2 in, 2 out]
        n550 = Bundle By Name(cluster=T75 {"Message"="", "Message Data"=variant} ("element"), "Message Data"="Mono1 Cut - Footswitch", "Message"="Mono1 Cut - Footswitch Activate Port") -> (w1323:T75)
        n551 = Enqueue Element(queue=w1320, element=w1323) -> (error out=w1321:errorcluster)  [unwired: 2 in, 2 out]
      }
      event "Mono1 Coag - Footswitch": Value Change {
        # "Turn power ON or OFF on MONO2 Coag Port"
        n552 = event-data() -> ()  [unwired: 1 in, 1 out]
        n553 = case shown="False" "Mono1 Coag - Footswitch" {
          tunnel: ["Deactivate Coag" ("Message") "Activate Coag" ("Message")] -> w1328
          frame True {
          }
          frame False {
          }
        }
        n554 = property on="Mono1 Coag - Footswitch" class="Bool (strict)"("BoolText.Text"=w1328) -> ()  [unwired: 2 in, 2 out]
        n555 = Bundle By Name(cluster=T75 {"Message"="", "Message Data"=variant} ("element"), "Message Data"="Mono1 Coag - Footswitch", "Message"="Mono1 Coag - Footswitch Activate Port") -> (w1334:T75)
        n556 = Enqueue Element(queue=w1331, element=w1334) -> (error out=w1332:errorcluster)  [unwired: 2 in, 2 out]
      }
      event "Mono2 Cut - Footswitch": Value Change {
        # "Turn power ON or OFF on MONO2 Coag Port"
        n557 = event-data() -> ()  [unwired: 1 in, 1 out]
        n558 = case shown="False" "Mono2 Cut - Footswitch" {
          tunnel: ["Deactivate Cut" ("Message") "Activate Cut" ("Message")] -> w1339
          frame True {
          }
          frame False {
          }
        }
        n559 = property on="Mono2 Cut - Footswitch" class="Bool (strict)"("BoolText.Text"=w1339) -> ()  [unwired: 2 in, 2 out]
        n560 = Bundle By Name(cluster=T75 {"Message"="", "Message Data"=variant} ("element"), "Message Data"="Mono2 Cut - Footswitch", "Message"="Mono2 Cut - Footswitch Activate Port") -> (w1345:T75)
        n561 = Enqueue Element(queue=w1342, element=w1345) -> (error out=w1343:errorcluster)  [unwired: 2 in, 2 out]
      }
      event "Mono2 Coag - Footswitch": Value Change {
        # "Turn power ON or OFF on MONO2 Coag Port"
        n562 = event-data() -> ()  [unwired: 1 in, 1 out]
        n563 = case shown="False" "Mono2 Coag - Footswitch" {
          tunnel: ["Deactivate Coag" ("Message") "Activate Coag" ("Message")] -> w1350
          frame True {
          }
          frame False {
          }
        }
        n564 = property on="Mono2 Coag - Footswitch" class="Bool (strict)"("BoolText.Text"=w1350) -> ()  [unwired: 2 in, 2 out]
        n565 = Bundle By Name(cluster=T75 {"Message"="", "Message Data"=variant} ("element"), "Message Data"="Mono2 Coag - Footswitch", "Message"="Mono2 Coag - Footswitch Activate Port") -> (w1356:T75)
        n566 = Enqueue Element(queue=w1353, element=w1356) -> (error out=w1354:errorcluster)  [unwired: 2 in, 2 out]
      }
      event "Mono2 Triverse - Footswitch": Value Change {
        # "Turn power ON or OFF on MONO2 Coag Port"
        n567 = event-data() -> ()  [unwired: 1 in, 1 out]
        n568 = case shown="False" "Mono2 Triverse - Footswitch" {
          tunnel: ["Deactivate" ("Message") "Activate" ("Message")] -> w1361
          frame True {
          }
          frame False {
          }
        }
        n569 = property on="Mono2 Triverse - Footswitch" class="Bool (strict)"("BoolText.Text"=w1361) -> ()  [unwired: 2 in, 2 out]
        n570 = Bundle By Name(cluster=T75 {"Message"="", "Message Data"=variant} ("element"), "Message Data"="Mono2 Triverse - Footswitch", "Message"="Mono2 Triverse - Footswitch Activate Port") -> (w1367:T75)
        n571 = Enqueue Element(queue=w1364, element=w1367) -> (error out=w1365:errorcluster)  [unwired: 2 in, 2 out]
      }
      event "Bipolar - Footswitch": Value Change {
        # "Turn power ON or OFF on MONO2 Coag Port"
        n572 = event-data() -> ()  [unwired: 1 in, 1 out]
        n573 = case shown="True" "Bipolar - Footswitch" {
          tunnel: ["Deactivate" ("Message") "Activate" ("Message")] -> w1373
          frame True {
          }
          frame False {
          }
        }
        n574 = property on="Bipolar - Footswitch" class="Bool (strict)"("BoolText.Text"=w1373) -> ()  [unwired: 2 in, 2 out]
        n575 = Bundle By Name(cluster=T75 {"Message"="", "Message Data"=variant} ("element"), "Message Data"="Bipolar - Footswitch", "Message"="Bipolar - Footswitch Activate Port") -> (w1378:T75)
        n576 = Enqueue Element(queue=w1375, element=w1378) -> (error out=w1376:errorcluster)  [unwired: 2 in, 2 out]
      }
      event "Ligasure - Bipolar Footswitch": Value Change {
        # "Turn power ON or OFF on MONO2 Coag Port"
        n577 = event-data() -> ()  [unwired: 1 in, 1 out]
        n578 = Bundle By Name(cluster=T75 {"Message"="", "Message Data"=variant} ("element"), "Message Data"="Ligasure - Bipolar Footswitch", "Message"="Lig Bipolar - Footswitch Activate Port") -> (w1388:T75)
        n579 = Enqueue Element(queue=w1385, element=w1388) -> (error out=w1386:errorcluster)  [unwired: 2 in, 2 out]
      }
      event "Ligasure - Seal Footswitch": Value Change {
        # "Turn power ON or OFF on MONO2 Coag Port"
        n580 = event-data() -> ()  [unwired: 1 in, 1 out]
        n581 = Bundle By Name(cluster=T75 {"Message"="", "Message Data"=variant} ("element"), "Message Data"="Ligasure - Seal Footswitch", "Message"="Lig Seal - Footswitch Activate Port") -> (w1396:T75)
        n582 = Enqueue Element(queue=w1393, element=w1396) -> (error out=w1394:errorcluster)  [unwired: 2 in, 2 out]
      }
      event "Ligasure - Cut Footswitch": Value Change {
        # "Turn power ON or OFF on MONO2 Coag Port"
        n583 = event-data() -> ()  [unwired: 1 in, 1 out]
        n584 = Bundle By Name(cluster=T75 {"Message"="", "Message Data"=variant} ("element"), "Message Data"="Ligasure - Cut Footswitch", "Message"="Lig Cut - Footswitch Activate Port") -> (w1404:T75)
        n585 = Enqueue Element(queue=w1401, element=w1404) -> (error out=w1402:errorcluster)  [unwired: 2 in, 2 out]
      }
      event "Ligasure - Coag Footswitch": Value Change {
        # "Turn power ON or OFF on MONO2 Coag Port"
        n586 = event-data() -> ()  [unwired: 1 in, 1 out]
        n587 = Bundle By Name(cluster=T75 {"Message"="", "Message Data"=variant} ("element"), "Message Data"="Ligasure - Coag Footswitch", "Message"="Lig Coag - Footswitch Activate Port") -> (w1412:T75)
        n588 = Enqueue Element(queue=w1409, element=w1412) -> (error out=w1410:errorcluster)  [unwired: 2 in, 2 out]
      }
      event Value Change {
        # "Turn power level down on MONO1 Cut Port"
        n589 = event-data() -> ()  [unwired: 1 in, 1 out]
        n590 = Bundle By Name(cluster=T75 {"Message"="", "Message Data"=variant} ("element"), "Message Data"="Mono1 Cut minus", "Message"="Mono1 Cut Decrease Power") -> (w1420:T75)
        n591 = Enqueue Element(queue=w1417, element=w1420) -> (error out=w1418:errorcluster)  [unwired: 2 in, 2 out]
      }
      event Value Change {
        # "Turn power level down on MONO2 Cut Port"
        n592 = event-data() -> ()  [unwired: 1 in, 1 out]
        n593 = Bundle By Name(cluster=T75 {"Message"="", "Message Data"=variant} ("element"), "Message Data"="Mono2 Cut minus", "Message"="Mono2 Cut Decrease Power") -> (w1428:T75)
        n594 = Enqueue Element(queue=w1425, element=w1428) -> (error out=w1426:errorcluster)  [unwired: 2 in, 2 out]
      }
      event Value Change {
        # "Turn power level down on MONO1 Coag Port"
        n595 = event-data() -> ()  [unwired: 1 in, 1 out]
        n596 = Bundle By Name(cluster=T75 {"Message"="", "Message Data"=variant} ("element"), "Message Data"="Mono1 Coag minus", "Message"="Mono1 Coag Decrease Power") -> (w1436:T75)
        n597 = Enqueue Element(queue=w1433, element=w1436) -> (error out=w1434:errorcluster)  [unwired: 2 in, 2 out]
      }
      event Value Change {
        # "Turn power level down on MONO2 Coag Port"
        n598 = event-data() -> ()  [unwired: 1 in, 1 out]
        n599 = Bundle By Name(cluster=T75 {"Message"="", "Message Data"=variant} ("element"), "Message Data"="Mono2 Coag minus", "Message"="Mono2 Coag Decrease Power") -> (w1444:T75)
        n600 = Enqueue Element(queue=w1441, element=w1444) -> (error out=w1442:errorcluster)  [unwired: 2 in, 2 out]
      }
      event Value Change {
        # "Turn power level down on Bipolar Port"
        n601 = event-data() -> ()  [unwired: 1 in, 1 out]
        n602 = Bundle By Name(cluster=T75 {"Message"="", "Message Data"=variant} ("element"), "Message Data"="Bipolar minus", "Message"="Bipolar Decrease Power") -> (w1452:T75)
        n603 = Enqueue Element(queue=w1449, element=w1452) -> (error out=w1450:errorcluster)  [unwired: 2 in, 2 out]
      }
      event Value Change {
        # "Turn power level up on MONO1 Cut Port"
        n604 = event-data() -> ()  [unwired: 1 in, 1 out]
        n605 = Bundle By Name(cluster=T75 {"Message"="", "Message Data"=variant} ("element"), "Message Data"="Mono1 Cut plus", "Message"="Mono1 Cut Increase Power") -> (w1460:T75)
        n606 = Enqueue Element(queue=w1457, element=w1460) -> (error out=w1458:errorcluster)  [unwired: 2 in, 2 out]
      }
      event Value Change {
        # "Turn power level up on MONO2 Cut Port"
        n607 = event-data() -> ()  [unwired: 1 in, 1 out]
        n608 = Bundle By Name(cluster=T75 {"Message"="", "Message Data"=variant} ("element"), "Message Data"="Mono2 Cut plus", "Message"="Mono2 Cut Increase Power") -> (w1468:T75)
        n609 = Enqueue Element(queue=w1465, element=w1468) -> (error out=w1466:errorcluster)  [unwired: 2 in, 2 out]
      }
      event Value Change {
        # "Turn power level up on MONO1 Coag Port"
        n610 = event-data() -> ()  [unwired: 1 in, 1 out]
        n611 = Bundle By Name(cluster=T75 {"Message"="", "Message Data"=variant} ("element"), "Message Data"="Mono1 Coag plus", "Message"="Mono1 Coag Increase Power") -> (w1476:T75)
        n612 = Enqueue Element(queue=w1473, element=w1476) -> (error out=w1474:errorcluster)  [unwired: 2 in, 2 out]
      }
      event Value Change {
        # "Turn power level up on MONO2 Coag Port"
        n613 = event-data() -> ()  [unwired: 1 in, 1 out]
        n614 = Bundle By Name(cluster=T75 {"Message"="", "Message Data"=variant} ("element"), "Message Data"="Mono2 Coag plus", "Message"="Mono2 Coag Increase Power") -> (w1484:T75)
        n615 = Enqueue Element(queue=w1481, element=w1484) -> (error out=w1482:errorcluster)  [unwired: 2 in, 2 out]
      }
      event Value Change {
        # "Turn power level up on Bipolar Port"
        n616 = event-data() -> ()  [unwired: 1 in, 1 out]
        n617 = Bundle By Name(cluster=T75 {"Message"="", "Message Data"=variant} ("element"), "Message Data"="Bipolar plus", "Message"="Bipolar Increase Power") -> (w1492:T75)
        n618 = Enqueue Element(queue=w1489, element=w1492) -> (error out=w1490:errorcluster)  [unwired: 2 in, 2 out]
      }
      event Value Change {
        # "Change mode on MONO1 Cut Port"
        n619 = event-data() -> ()  [unwired: 1 in, 1 out]
        n620 = Bundle By Name(cluster=T75 {"Message"="", "Message Data"=variant} ("element"), "Message Data"="Mono1 Cut Enum", "Message"="Mono1 Cut Mode") -> (w1500:T75)
        n621 = Enqueue Element(queue=w1497, element=w1500) -> (error out=w1498:errorcluster)  [unwired: 2 in, 2 out]
      }
      event Value Change {
        # "Change mode on MONO2 Cut Port"
        n622 = event-data() -> ()  [unwired: 1 in, 1 out]
        n623 = Bundle By Name(cluster=T75 {"Message"="", "Message Data"=variant} ("element"), "Message Data"="Mono2 Cut Enum", "Message"="Mono2 Cut Mode") -> (w1508:T75)
        n624 = Enqueue Element(queue=w1505, element=w1508) -> (error out=w1506:errorcluster)  [unwired: 2 in, 2 out]
      }
      event Value Change {
        # "Change mode on MONO1 Coag Port"
        n625 = event-data() -> ()  [unwired: 1 in, 1 out]
        n626 = Bundle By Name(cluster=T75 {"Message"="", "Message Data"=variant} ("element"), "Message Data"="Mono1 Coag Enum", "Message"="Mono1 Coag Mode") -> (w1516:T75)
        n627 = Enqueue Element(queue=w1513, element=w1516) -> (error out=w1514:errorcluster)  [unwired: 2 in, 2 out]
      }
      event Value Change {
        # "Change mode on MONO2 Coag Port"
        n628 = event-data() -> ()  [unwired: 1 in, 1 out]
        n629 = Bundle By Name(cluster=T75 {"Message"="", "Message Data"=variant} ("element"), "Message Data"="Mono2 Coag Enum", "Message"="Mono2 Coag Mode") -> (w1524:T75)
        n630 = Enqueue Element(queue=w1521, element=w1524) -> (error out=w1522:errorcluster)  [unwired: 2 in, 2 out]
      }
      event Value Change {
        # "Change mode on Bipolar Port"
        n631 = event-data() -> ()  [unwired: 1 in, 1 out]
        n632 = Bundle By Name(cluster=T75 {"Message"="", "Message Data"=variant} ("element"), "Message Data"="Bipolar Enum", "Message"="Bipolar Mode") -> (w1532:T75)
        n633 = Enqueue Element(queue=w1529, element=w1532) -> (error out=w1530:errorcluster)  [unwired: 2 in, 2 out]
      }
      event "Update Semi-Auto": Value Change {
        # "Update the command cluster"
        n634 = event-data() -> ()  [unwired: 1 in, 1 out]
        n635 = call "FT10_Semi-Auto Tester.vi"("Read/ Write"="Read/ Write", "Semi-Auto Cluster in"="Semi-Auto Cluster in", "Path"="Path") -> ("Semi-Auto Cluster out"=w1536:T48, "Semi-Auto 2-D Array out"=→"Semi-Auto 2-D Array out":T47)  [unwired: 6 in, 1 out]
      }
      event "Run Semi-Auto Commands": Value Change {
        n636 = event-data() -> ()  [unwired: 1 in, 1 out]
        n637 = for {
          tunnel: w1542 -> [w1545]
          tunnel: w1541 -> [w1544] mode=indexing
          n638 = call "FT10_Semi-Auto Parse Commands.vi"("Semi-Auto Cluster"=w1544) -> ("appended array"=w1543:T102[])  [unwired: 10 in]
          n639 = for {
            tunnel: w1545 -> [w1550]
            tunnel: w1543 -> [w1549] mode=indexing
            n640 = Unbundle By Name(w1549) -> ("Wait Time (ms)"=w1546:i32, "Message Data"=w1548:variant, "Message"=w1547:string)
            n641 = Wait (ms)(milliseconds to wait=w1546) -> ()  [unwired: 1 out]
            n642 = Bundle By Name(cluster=T75 {"Message"="", "Message Data"=variant} ("element"), "Message Data"=w1548, "Message"=w1547) -> (w1551:T75)
            n643 = Enqueue Element(queue=w1550, element=w1551) -> ()  [unwired: 2 in, 3 out]
          }
        }
      }
      event "Update Semi-Auto 2": Value Change {
        n644 = event-data() -> ()  [unwired: 1 in, 1 out]
        n645 = call "FT10_Semi-Auto 2 Tester.vi"("Read/ Write"="Read/ Write 2", "Semi-Auto 2 Cluster in"="Semi-Auto 2 Cluster in", "Path"="Path 2") -> ("Semi-Auto 2 Cluster out"=w1553:T56, "Semi-Auto 2-D Array out"=→"Semi-Auto 2-D Array out 2":T47)  [unwired: 6 in, 1 out]
      }
      event "Run Semi-Auto 2 Commands": Value Change {
        n646 = event-data() -> ()  [unwired: 1 in, 1 out]
        n647 = for {
          tunnel: w1562 -> [w1565]
          tunnel: w1560 -> [w1563] mode=indexing
          n648 = call "FT10_Semi-Auto 2 Parse Commands.vi"("Semi-Auto 2 Cluster in"=w1563) -> ("appended array"=w1564:T102[])  [unwired: 10 in]
          n649 = for {
            tunnel: w1565 -> [w1570]
            tunnel: w1564 -> [w1569] mode=indexing
            n650 = Unbundle By Name(w1569) -> ("Wait Time (ms)"=w1566:i32, "Message Data"=w1568:variant, "Message"=w1567:string)
            n651 = Wait (ms)(milliseconds to wait=w1566) -> ()  [unwired: 1 out]
            n652 = Bundle By Name(cluster=T75 {"Message"="", "Message Data"=variant} ("element"), "Message Data"=w1568, "Message"=w1567) -> (w1571:T75)
            n653 = Enqueue Element(queue=w1570, element=w1571) -> ()  [unwired: 2 in, 3 out]
          }
        }
      }
      event Value Change {
        w1574 = TRUE
        # "Stop the VI."
        # "Enqueue an \"Exit\" message. Note that the Enqueue Element At Opposite End function is used to place this priority \"Exit\" message at the front of the queue ahead of all other messages."
        n654 = event-data() -> ()  [unwired: 1 in, 1 out]
        n655 = Enqueue Element At Opposite End(queue=w1576, element=T75 {"Message"="Exit", "Message Data"=variant}) -> (error out=w1578:errorcluster)  [unwired: 2 in, 2 out]
      }
      event Panel Close? {
        # "Stop the VI."
        # "Enqueue an \"Exit\" message. Note that the Enqueue Element At Opposite End function is used to place this priority \"Exit\" message at the front of the queue ahead of all other messages."
        n656 = event-data() -> ()  [unwired: 1 in, 1 out]
        n657 = Enqueue Element At Opposite End(queue=w1581, element=T75 {"Message"="Exit", "Message Data"=variant}) -> (error out=w1584:errorcluster)  [unwired: 2 in, 2 out]
        n658 = event-data() -> ()  [unwired: 2 in, 1 out]
      }
    }
  }
  n659 = while {
    tunnel: w1 -> [w1585]
    stop <- w1586 stop-if-true
    n660 = global write "Abort Auto Test Global.vi" "Abort Auto Test"("Abort Auto Test") -> ()
    n661 = Or(x=w1585, y="Stop Button") -> (x .or. y?=w1586:bool)
  }
  n662 = Release Queue(queue=w6, error in (no error)=w7) -> (error out=w5:errorcluster)  [unwired: 1 in, 2 out]
  n663 = Merge Errors(w27, w28, w5) -> (w16:errorcluster)
  n664 = call "FT10_Stop Notifier.vi"("Selector"=Config_Stop_Notifier_Enum."Close", "error in (no error)"=w16) -> ("error out"=w15:errorcluster)  [unwired: 8 in, 1 out]
  n665 = call <vilib>:"Simple Error Handler.vi"("error in (no error)"=w15) -> ()  [unwired: 4 in, 5 out]
